vi "Orbitron2Websdr_MainApp_20032021.vi"() -> ()   [LabVIEW 2021]
uses:
  FHASOF_Groundstationsoftware/D/LabVIEW 2021/FHASOF_Groundstationsoftware/Multitrack.llb/Window Rectangle.ctl
  <vilib>/Utility/error.llb/whitespace.ctl
  <vilib>/Platform/TimedLoop/XDataNode/timing_clust.ctl
  <vilib>/Platform/TimedLoop/XDataNode/nitl_modes.ctl
  <vilib>/Platform/TimedLoop/XDataNode/wakeup.ctl
  <vilib>/Utility/error.llb/DialogType.ctl
  <vilib>/platform/TimedLoop/XDataNode/XDataNode.xnode
  <vilib>/Platform/TimedLoop/XDataNode/XDNodeRunTimeDep.lvlib
  <vilib>/Platform/browser.llb/Open URL in Default Browser (string).vi
panel:
  out "MaOps":bool
  out "error out 3":errorcluster
  out "error out 2":errorcluster
  out "path 3":path
  in  "Tab Control":T1(tab)
  out "Satellite Name":string
  in  "FocusCheck":bool
  in  "load":bool
  in  "Start browser":bool
  in  "preferences":bool
  in  "Stop_Button":bool
  out "Title 2":string="WebSDR Cat Control"
  in  "cw":bool
  in  "FocusWebSDR":bool
  in  "OpenWebSDR":bool
  in  "WebPages":u16(ring)=2 items=["IJsselstein, the Netherlands, JO22MA62KJ.", "IS0GRB VHF WebSDR Receiver IS0GRB / south sartinian iland", "Novovoronezh WebSDR WX"]
  in  "AddWebSDR":bool
  in  "Truncate Left digits":i32 caption="kHz"
  in  "Stop Cat Control":bool
  in  "Cat Control":bool
  in  "TaskList_Button":bool
  in  "processes Box":string(combo)="WebSDR on R3KEE in Novovoronezh - Google Chrome"
  out "Azimuth":string caption="°"
  out "Elevation":string caption="°"
  out "Downlink Freq.":string caption="KHz"
  in  "Downlink Freq. Man.":dbl=137100.0 caption="kHz" format="%#_6f"
  in  "ManualLatch":bool
  in  "Radio Mode":bool=TRUE
  in  "Type of DN":string
  in  "Downlink corr.":dbl(knob) scale=-100.0..100.0
  in  "USB":bool
  in  "LSB":bool
  in  "AM":bool
  in  "FM":bool
  in  "EditWebSDR":bool
  in  "DeleteWebSDR":bool
  out "Mode":string="Radio Manual mode"
  in  "Path of the webbrowser to start WebSDR":path=path "C:/Program Files/Google/Chrome/Application/chrome.exe"
  in  "goback_button":bool
  in  "Cancel Edit 2":bool
  out "data":string caption="DDE Message"
  in  "Sampling interval":u32=1000 caption="[ms]"
  in  "Load_button":bool
  in  "Cancel load":bool
  in  "Load controlfile":path=path "C:/Users/Setup/Documents/LabVIEW 2021"
  in  "Downlink corr.":string="0,000000"
  in  "Title":string="Add a new WebSDR database item"
  in  "Cancel Edit":bool
  in  "Edit_Button":bool
  in  "WebSDR Location / Name":string="Novovoronezh WebSDR WX"
  in  "Cancel Add":bool
  in  "Add_Button":bool
  in  "WebSDR URL":string="http://websdr.vrn.ru:8901/"
  in  "Window title":string="WebSDR on R3KEE in Novovoronezh - Google Chrome"
  in  "Truncate digits":string="2"
  out "Title 3":string="WebSDR Cat Control"
  in  "WebSDRDB":string[][](array[string])=[["IJsselstein, the Netherlands, JO22MA62KJ.", "WebSDR on Gerbrandy Tower in IJsselstein, NL - Google Chrome", "http://websdr.pi1utr.ampr.org:8901/", "0"], ["IS0GRB VHF WebSDR Receiver IS0GRB / south sartinian iland", "IS0GRB VHF WebSDR Receiver - Google Chrome", "http://websdr.is0grb.it:8902/", "2"], ["Novovoronezh WebSDR WX", "WebSDR on R3KEE in Novovoronezh - Google Chrome", "http://websdr.vrn.ru:8901/", "2"]]
  in  "Numeric":i32
  out "error out":errorcluster={"status"=FALSE, "code"=0, "source"="Get Window ID.vi"}
  out "Active Processses":string
  out "standard error":string
  out "standard output":string
  out "window rect 2":T2={"left"=-5, "top"=-564, "right"=1089, "bottom"=-2}
  in  "window names":string[](array[string])=["Orbitron 3.71", "WebSDR on R3KEE in Novovoronezh - Google Chrome", "Mydde", "RX-SSTV", "Task-Manager", "Einstellungen", "Einstellungen", "VIPM Service", "Microsoft Text Input Application", "Mail", "Posteingang – Hotmail ?- Mail", "Orbitron2Websdr_Win10Build", "RX-SSTV", "Program Manager", "LabVIEW"]
  in  "kill":bool
  in  "StopCatProgramatically":bool
  out "shutdown in":bool
  in  "iterCompleted":bool
  in  "slave4Killed":bool
  in  "slave3Killed":bool
  in  "slave1Killed":bool
  out "Elapsed Time (s)":dbl=3.000234603881836
  out "path 2":path
  out "path 4":path=path "C:/Users/Setup/Documents/LabVIEW 2021/Orbitron2Websdr_MainApp_20032021.ctr"
  out "path":path=path "C:/Users/Setup/Documents/LabVIEW 2021/Orbitron2Websdr_MainApp_20032021.ctr"
  out "concatenated string":string="Orbitron2Websdr_MainApp_20032021\\"
  out "string":string="C:\\Users\\Setup\\Documents\\LabVIEW 2021\\Orbitron2Websdr_MainApp_20032021.ctr"
  out "Parent Directory (+ Relative)":path=path "C:/Users/Setup/Documents/LabVIEW 2021"
  in  "dont write":bool
  in  "Interrupt":bool
  in  "AppName":string="WebSDR1"
  # "For Orbitron 3.71 MyDDE-Driver"
  # "To start WebSDR, you need a Webbrowser. We had good experiences using Firefox, so we selected Firefox as the default browser. If you want to start your WebSDR sessions with another browser,just select the executable of your preferred browser here:"
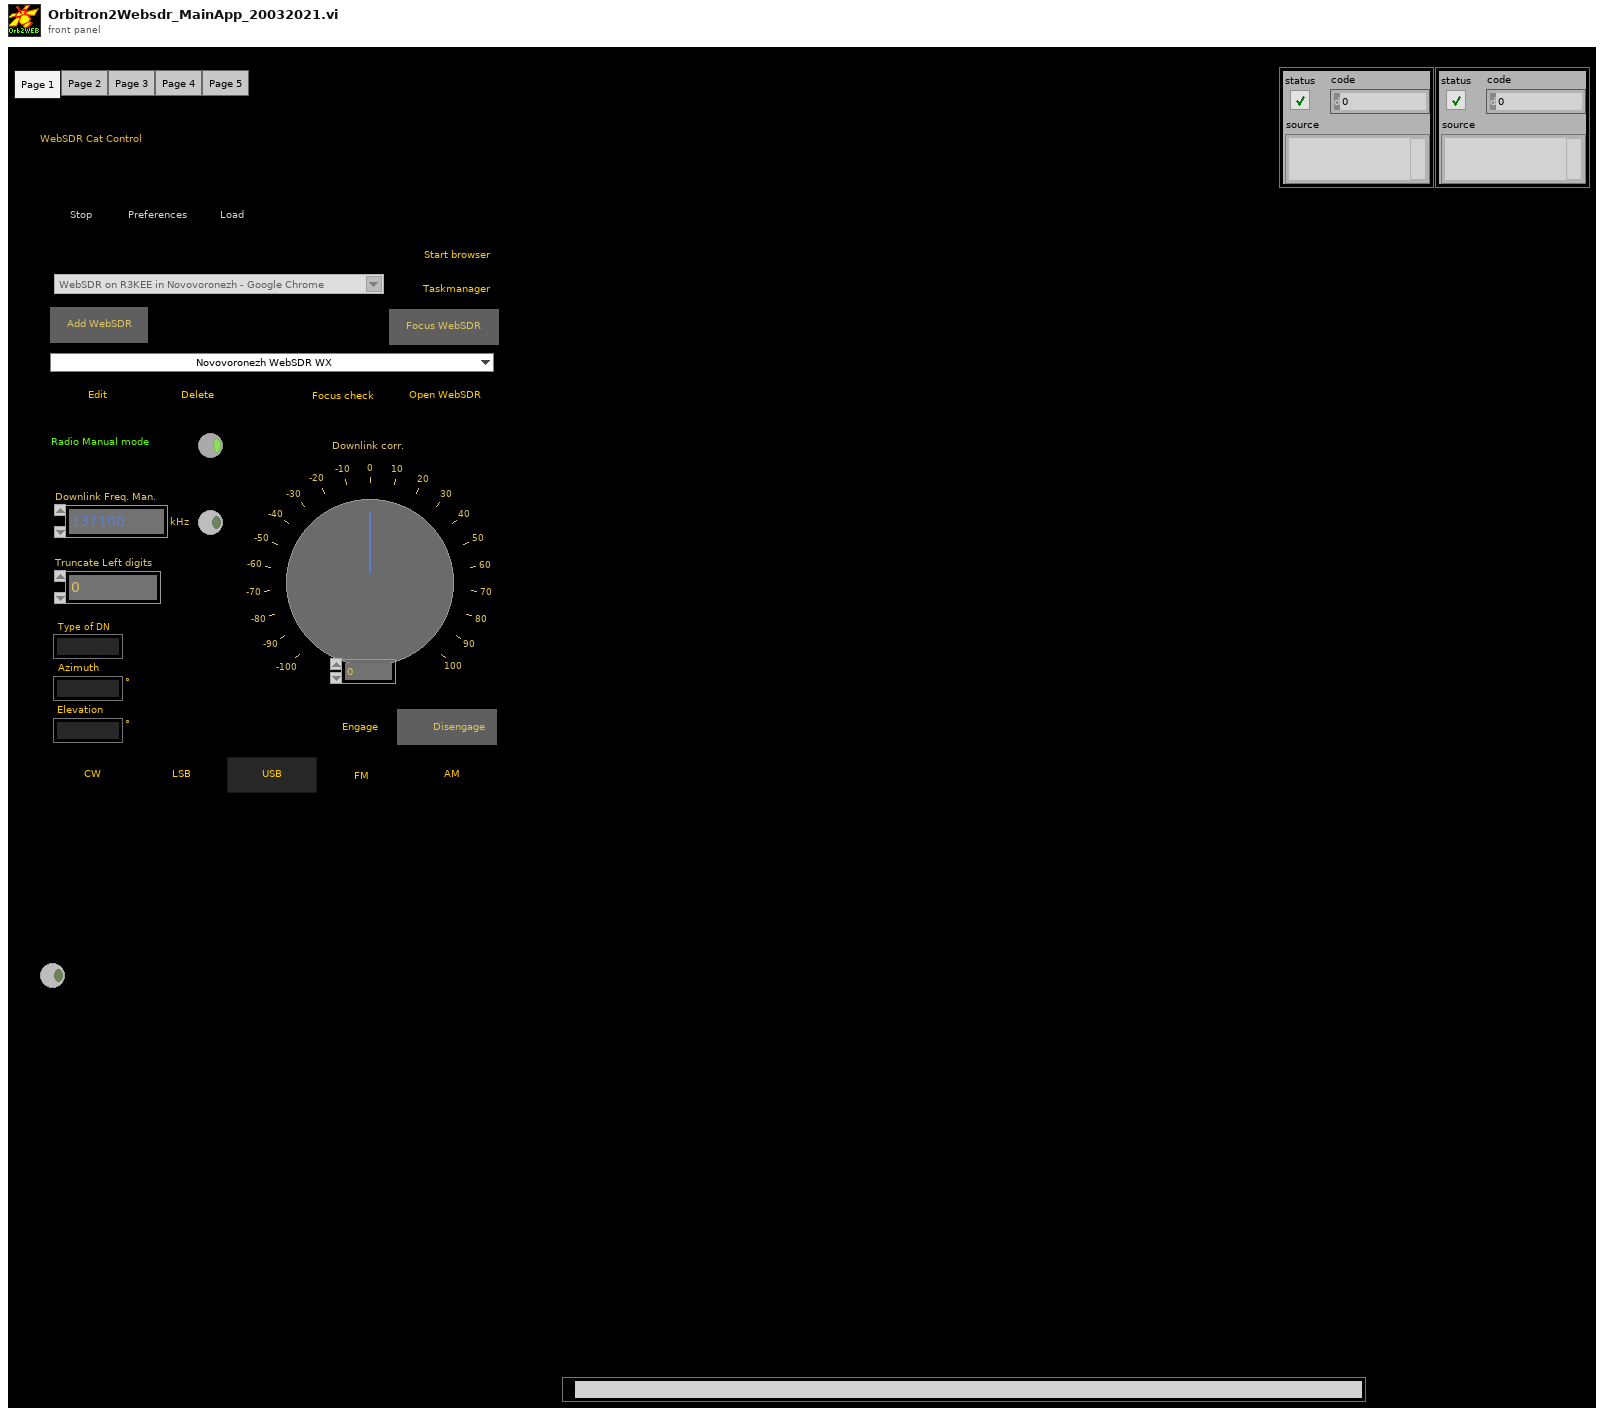
[diagram p1: front panel]
types:
  T1 = enum32{"Page 1", "Page 2", "Page 3", "Page 4", "Page 5"}
  T2 = typedef "Window Rectangle.ctl" = cluster{"left":i16, "top":i16, "right":i16, "bottom":i16}
  T3 = enum8{"Enabled", "Disabled", "Disabled and Grayed Out"}
  T4 = enum16{"Get Number of Tasks", "Get Window Info", "Get Window Names"}
  T5 = cluster{"number of windows":i32, "total names length":u32, "number of tasks found":i32, "window handles":u32[], "process ID":u32}
  T6 = typedef "Window Refnum" = refnum<k1>
  T7 = typedef "XDNodeRunTimeDep.lvlib/timing_clust.ctl" = cluster{"Expected End [f-1]":u64, "Actual End [f-1]":u64, "Finished Late? [f-1]":bool, "Expected End [i-1]":u64, "Actual End [i-1]":u64, "Finished Late? [i-1]":bool, "Expected Start [i]":u64, "Actual Start [i]":u64, "Expected Start [f]":u64, "Actual Start [f]":u64, "Source Name":string, "Structure Name":string, "Period":i64, "Deadline":i64, "Offset":i64, "Start":i64, "Priority":i32, "Timeout":i32, "Mode":T8, "Wakeup Reason":T9, "Error":errorcluster, "Source Type":string, "Secondary Source Type":string, "Global End Time":u64, "Global Start Time":u64, "Frame Duration":u64, "Iteration Duration":u64, "Assigned CPU":i32, "I/O Scan Engine Mode":u32}
  T8 = typedef "XDNodeRunTimeDep.lvlib/nitl_modes.ctl" = enum32{"No Change", "Process missed periods, maintain original phase", "Discard missed periods, maintain original phase", "Process missed periods, ignore original phase", "Discard missed periods, ignore original phase"}
  T9 = typedef "XDNodeRunTimeDep.lvlib/wakeup.ctl" = enum32{"Normal", "Aborted", "Asynchronous wakeup", "Timing source error", "Timed loop error", "Timeout"}
  T10 = typedef "DialogType.ctl" = u16
  T11 = typedef "whitespace.ctl" = u16
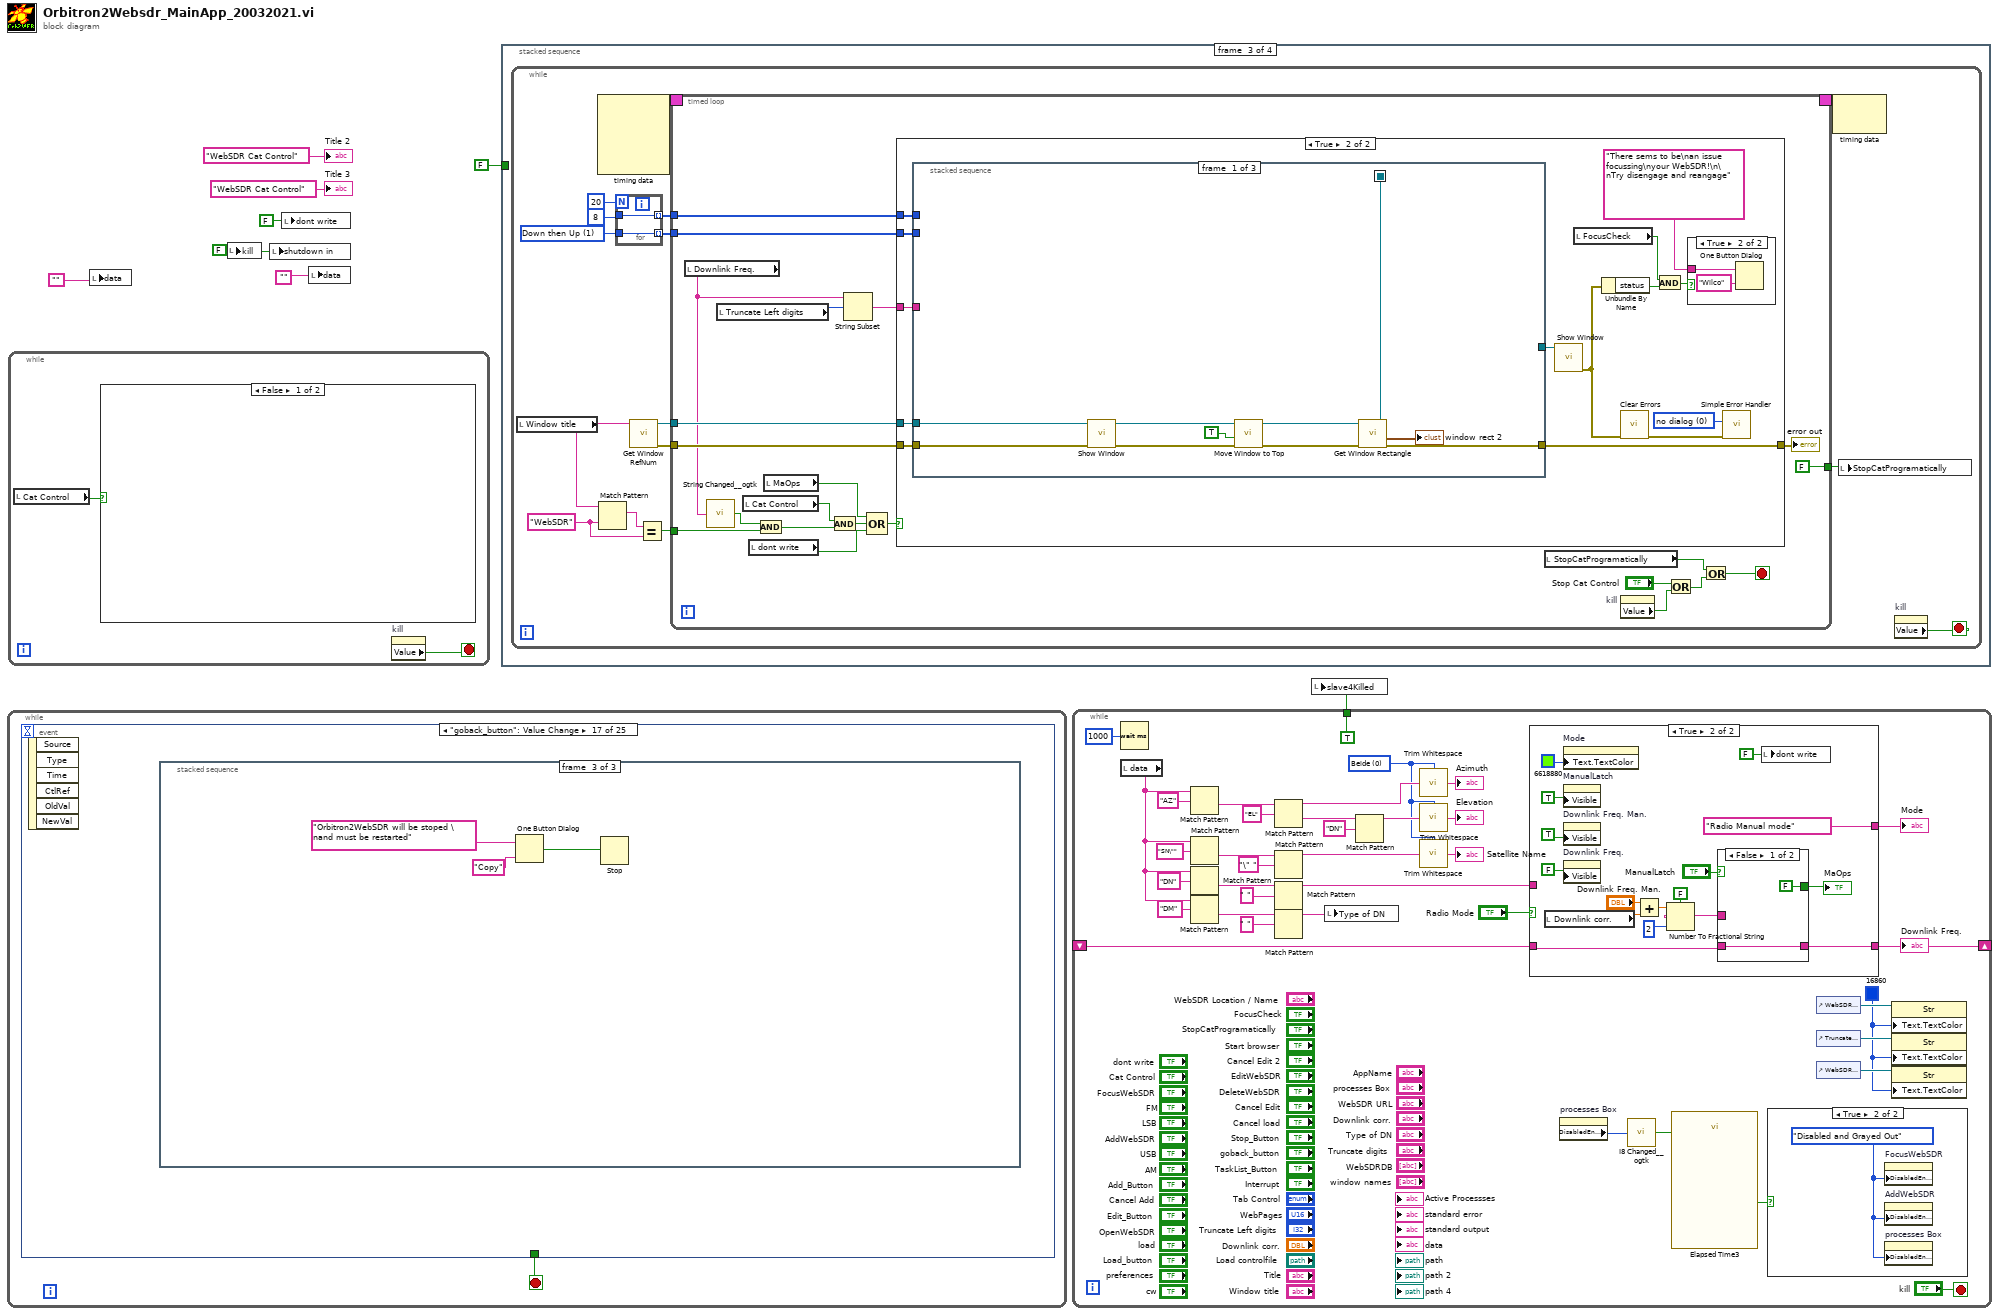
[diagram p0: block diagram]
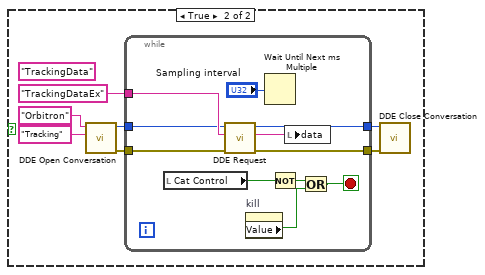
[diagram p2: hidden frame]
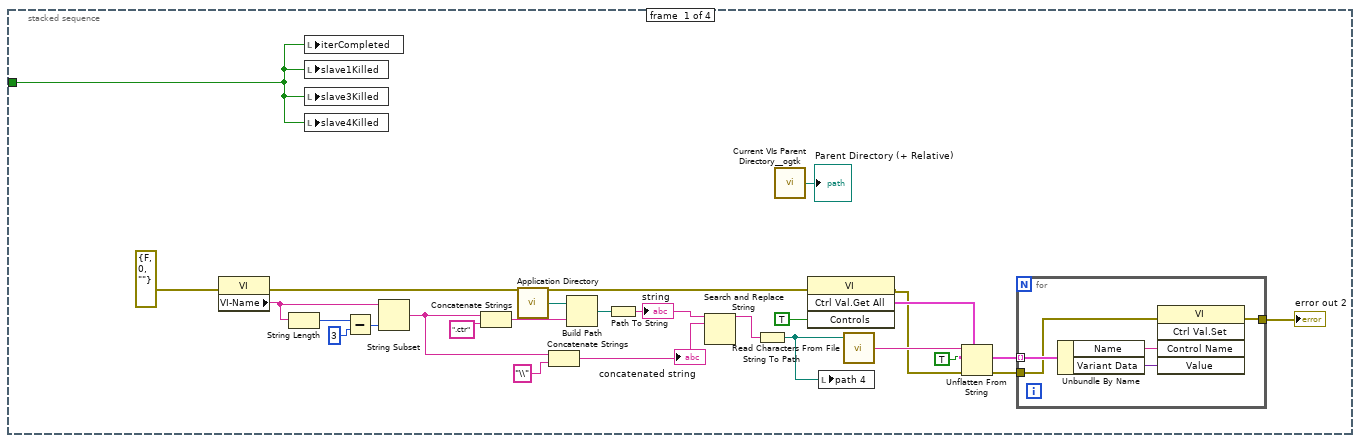
[diagram p3: hidden frame]
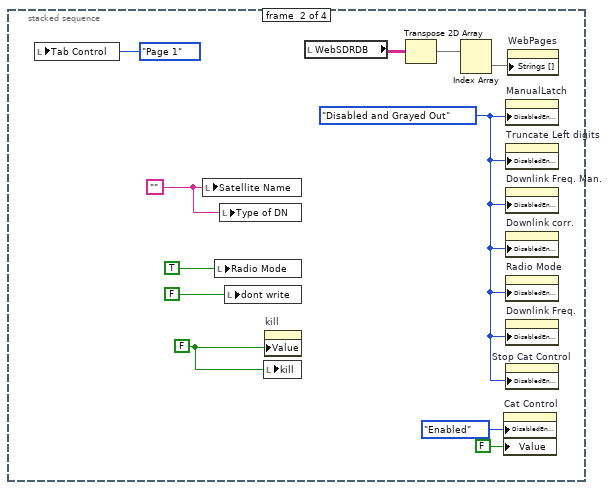
[diagram p4: hidden frame]
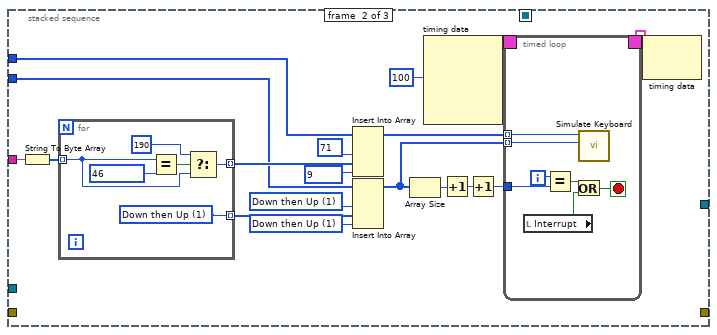
[diagram p7: hidden frame]
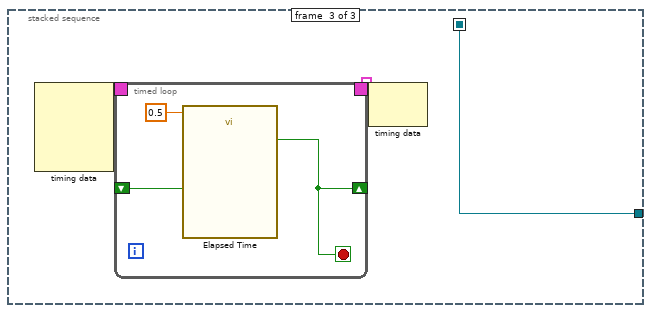
[diagram p8: hidden frame]
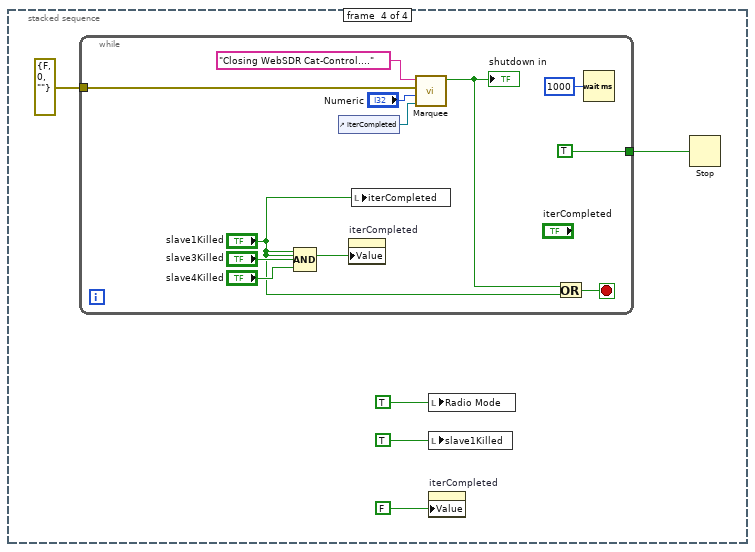
[diagram p9: hidden frame]
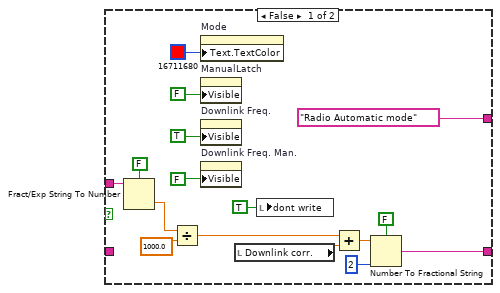
[diagram p11: hidden frame]
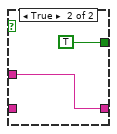
[diagram p12: hidden frame]
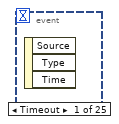
[diagram p13: hidden frame]
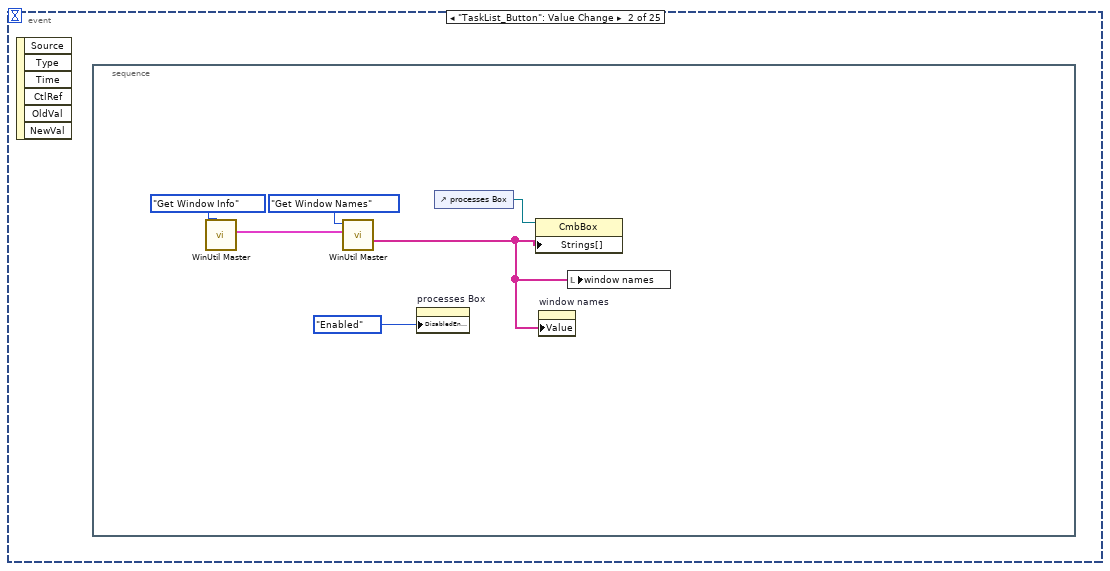
[diagram p14: hidden frame]
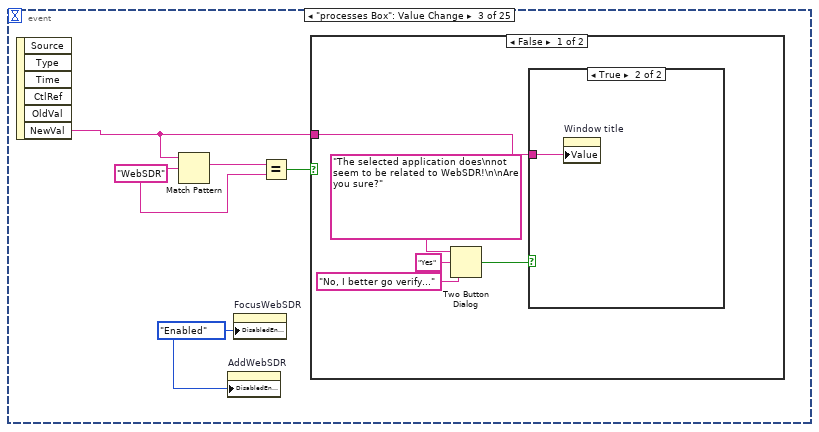
[diagram p15: hidden frame]
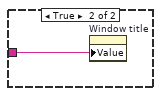
[diagram p17: hidden frame]
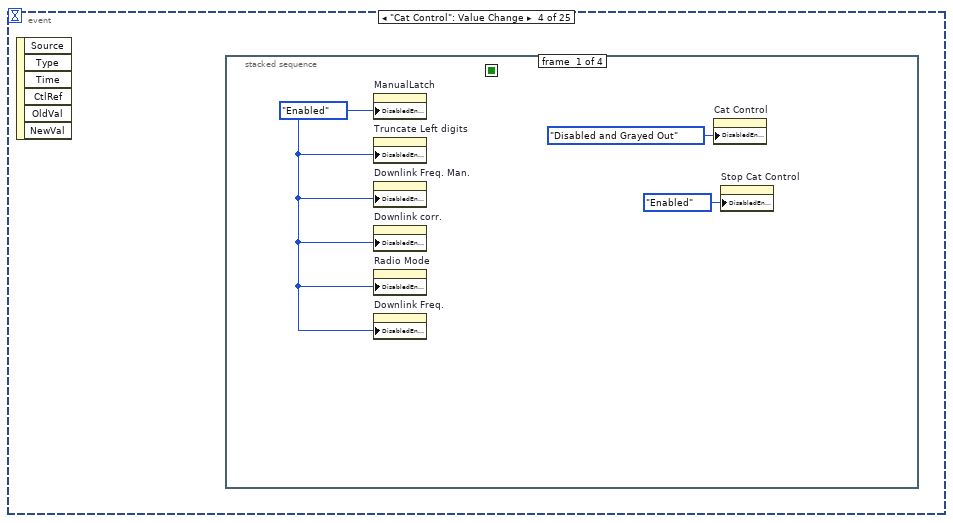
[diagram p18: hidden frame]
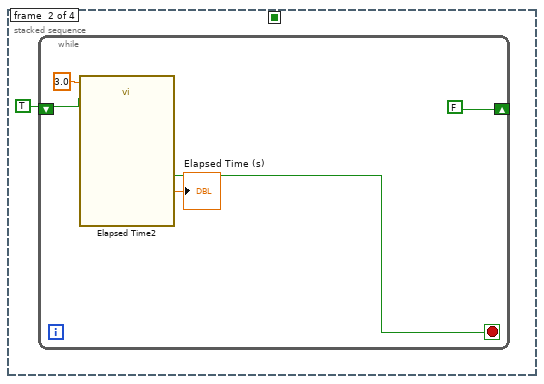
[diagram p19: hidden frame]
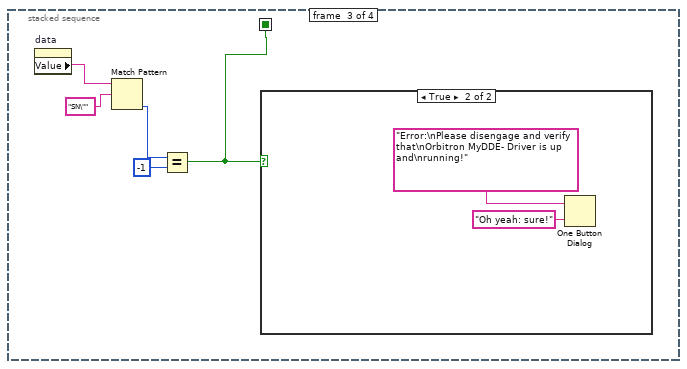
[diagram p20: hidden frame]
diagram:
  w6 = FALSE ("kill")
  n1 = while {
    stop <- w9 stop-if-true
    n2 = event shown="[16] \"goback_button\": Value Change" {
      selector: _ -> [_ _ _ _ _ _ _ _ _ _ _ _ _ _ _ _ _ _ _ _ _ _ _ _ _]
      dyn-events: _ -> [_ _ _ _ _ _ _ _ _ _ _ _ _ _ _ _ _ _ _ _ _ _ _ _ _]
      timeout: _ -> [_ _ _ _ _ _ _ _ _ _ _ _ _ _ _ _ _ _ _ _ _ _ _ _ _]
      tunnel: [_ _ _ _ w45 w95 _ _ _ _ _ _ _ _ _ _ _ _ _ _ _ _ _ _ _] -> w9
      event Timeout {
        n3 = event-data() -> ()  [unwired: 1 in, 3 out]
      }
      event "TaskList_Button": Value Change {
        n4 = event-data() -> ()  [unwired: 1 in, 6 out]
        n5 = stacked-sequence {
          frame #0 {
            n6 = call "WinUtil Master.vi"("function"=T4."Get Window Info") -> ("window enumeration info out"=w14:T5)  [unwired: 4 in, 2 out]
            n7 = call "WinUtil Master.vi"("window enumeration info in"=w14, "function"=T4."Get Window Names") -> ("window names"=w11:string[])  [unwired: 3 in, 2 out]
            n8 = property on="processes Box" class="CmbBox"("DisabledEnum"=T3."Enabled" ("Disabled")) -> ()  [unwired: 2 in, 2 out]
            n9 = control-ref of="processes Box"() -> (w15:refnum<vi>)
            n10 = property on="Property Node" class="CmbBox"(reference=w15, "Strings[]"=w11) -> ()  [unwired: 1 in, 2 out]
            n11 = property on="window names" class="Arr (strict)"("Value"=w11) -> ()  [unwired: 2 in, 2 out]
            n12 = local write "window names"(w11) -> ()
          }
        }
      }
      event "processes Box": Value Change {
        w17 = "WebSDR" ("Such-String")
        w20 = T3."Enabled" ("Disabled")
        n13 = event-data() -> ("NewVal"=w19:string)  [unwired: 1 in, 5 out]
        n14 = Match Pattern(string=w19, regular expression=w17) -> (match substring=w18:string)  [unwired: 1 in, 3 out]
        n15 = property on="AddWebSDR" class="Bool"("DisabledEnum"=w20) -> ()  [unwired: 2 in, 2 out]
        n16 = property on="FocusWebSDR" class="Bool"("DisabledEnum"=w20) -> ()  [unwired: 2 in, 2 out]
        n17 = Equal?(x=w18, y=w17) -> (x = y?=w16:bool)
        n18 = case shown="False" w16 {
          tunnel: w19 -> [w21 w27]
          frame False {
            n19 = Two Button Dialog(message="The selected application does\nnot seem to be related to WebSDR!\n\nAre you sure?", 1:"No, I better go verify..." ("F button name (\"Cancel\")"), 2:"Yes" ("T button name (\"OK\")")) -> (T button?=w22:bool)
            n20 = case shown="True" w22 {
              tunnel: w21 -> [_ w26]
              frame False {
              }
              frame True {
                n21 = property on="Window title" class="Str"("Value"=w26) -> ()  [unwired: 2 in, 2 out]
              }
            }
          }
          frame True {
            n22 = property on="Window title" class="Str"("Value"=w27) -> ()  [unwired: 2 in, 2 out]
          }
        }
      }
      event "Cat Control": Value Change {
        n23 = event-data() -> ()  [unwired: 1 in, 6 out]
        n24 = stacked-sequence {
          seq-local: [_ _ w38 _] -> [_ _ _ w44]
          frame #0 {
            w28 = T3."Enabled" ("Disabled")
            n25 = property on="ManualLatch" class="Bool"("DisabledEnum"=w28) -> ()  [unwired: 2 in, 2 out]
            n26 = property on="Truncate Left digits" class="DigNum (strict)"("DisabledEnum"=w28) -> ()  [unwired: 2 in, 2 out]
            n27 = property on="Downlink Freq. Man." class="DigNum (strict)"("DisabledEnum"=w28) -> ()  [unwired: 2 in, 2 out]
            n28 = property on="Downlink corr." class="Knob (strict)"("DisabledEnum"=w28) -> ()  [unwired: 2 in, 2 out]
            n29 = property on="Radio Mode" class="Bool (strict)"("DisabledEnum"=w28) -> ()  [unwired: 2 in, 2 out]
            n30 = property on="Downlink Freq." class="Str"("DisabledEnum"=w28) -> ()  [unwired: 2 in, 2 out]
            n31 = property on="Cat Control" class="Bool (strict)"("DisabledEnum"=T3."Disabled and Grayed Out" ("Disabled")) -> ()  [unwired: 2 in, 2 out]
            n32 = property on="Stop Cat Control" class="Bool"("DisabledEnum"=T3."Enabled" ("Disabled")) -> ()  [unwired: 2 in, 2 out]
          }
          frame #1 {
            n33 = while {
              shift-right: [FALSE] -> _
              shift-left: TRUE -> [w33]
              stop <- w35 stop-if-true
              n34 = call "Elapsed Time2"("Time Target (s)"=3.0, "Reset"=w33) -> ("Elapsed Time (s)"=→"Elapsed Time (s)":dbl, "Time has Elapsed"=w35:bool)  [unwired: 10 in, 6 out]
            }
          }
          frame #2 {
            n35 = property on="data" class="Str"() -> ("Value"=w37:string)  [unwired: 2 in, 2 out]
            n36 = Match Pattern(string=w37, regular expression="SN\"" ("Regulärer Ausdruck")) -> (offset past match=w40:i32)  [unwired: 1 in, 3 out]
            n37 = Equal?(x=w40, y=-1) -> (x = y?=w38:bool)
            n38 = case shown="True" w38 {
              frame False {
              }
              frame True {
                n39 = One Button Dialog(message="Error:\nPlease disengage and verify that\nOrbitron MyDDE- Driver is up and\nrunning!", button name ("OK")="Oh yeah: sure!") -> ()  [unwired: 1 out]
              }
            }
          }
          frame #3 {
            n40 = case shown="False" w44 {
              frame False {
                n41 = call "Display Message to User2"() -> ()  [unwired: 10 in, 2 out]
              }
              frame True {
              }
            }
          }
        }
      }
      event "Stop_Button": Value Change {
        n42 = event-data() -> ()  [unwired: 1 in, 6 out]
        n43 = stacked-sequence {
          tunnel: [_ _ w94] -> w45
          frame #0 {
            n44 = One Button Dialog(message="Ok WebSDR Cat Control\nwill be stoped!\nThis may take a while, \nso be a little bit patient!") -> ()  [unwired: 1 in, 1 out]
          }
          frame #1 {
            w55 = "websdrOrbitron" ("regular expression")
            n45 = property class="VI"() -> ("VI-Name"=w65:string)  [unwired: 2 in, 2 out]
            n46 = call "Current VIs Parent Directory__ogtk.vi"() -> ("Parent Directory (+ Relative)"=w49:path)  [unwired: 5 in]
            n47 = String Length(string=w65) -> (length=w63:i32)
            n48 = Subtract(x=w63, y=3) -> (x-y=w64:i32)
            n49 = String Subset(string=w65, length (rest)=w64) -> (substring=w82:string)  [unwired: 1 in]
            n50 = Concatenate Strings(w82, "*" ("string")) -> (w80:string)
            n51 = List Folder(path=w49, pattern=w80) -> (filenames=w81:string[])  [unwired: 2 in, 3 out]
            n52 = for {
              tunnel: w81 -> [w83] mode=indexing
              tunnel: w55 -> [w86]
              tunnel: [w85] -> w71 mode=indexing
              tunnel: [w83] -> _ mode=indexing
              n53 = Match Pattern(string=w83, regular expression=w86) -> (after substring=w84:string)  [unwired: 1 in, 3 out]
              n54 = Decimal String To Number(string=w84) -> (number=w85:i32)  [unwired: 2 in, 1 out]
            }
            n55 = Concatenate Strings(w82, ".ctr" ("String")) -> (w79:string)
            n56 = Build Path(base path=w49, name or relative path=w79) -> (appended path=w59:path)
            n57 = Array Max & Min(array=w71) -> (max value=w78:i32)  [unwired: 3 out]
            n58 = Concatenate Strings(w65, "\\" ("string")) -> (w62:string)
            n59 = Path To String(path=w59) -> (string=w60:string)
            n60 = Increment(x=w78) -> (x+1=w70:i32)
            n61 = Search and Replace String(input string=w60, search string=w62) -> (result string=w61:string)  [unwired: 6 in, 3 out]
            n62 = Format Value(format string="%03d", value (0)=w70) -> (output string=w69:string)  [unwired: 1 in]
            n63 = String To Path(string=w61) -> (path=w66:path)
            n64 = local write "path"(w66) -> ()
            n65 = Concatenate Strings(w55, w69) -> (w77:string)
            n66 = Concatenate Strings(w77, ".ctr" ("String")) -> (w72:string)
            n67 = invoke class="VI" method="Ctrl Val.Get All"("Controls"=TRUE ("controls")) -> ("Get All Control Values Variant"=w67:cluster{"Name":string, "Variant Data":variant}[])  [unwired: 3 in, 3 out]
            n68 = Build Path(base path=w49, name or relative path=w72) -> (appended path=w76:path)
            n69 = Concatenate Strings(w77, "\\" ("string")) -> (w73:string)
            n70 = Path To String(path=w76) -> (string=w75:string)
            n71 = Search and Replace String(input string=w75, search string=w73) -> (result string=w74:string)  [unwired: 6 in, 3 out]
            n72 = String To Path(string=w74) -> (path=w48:path)
            n73 = Flatten To String(anything=w67, prepend array or string size? (T)=TRUE) -> (data string=w68:string)  [unwired: 2 in, 2 out]
            n74 = stacked-sequence {
              tunnel: w66 -> [_ w89 _ w92 _]
              tunnel: w68 -> [w87 _ _ w91 _]
              tunnel: w48 -> [w88 _ _ _ _]
              frame #0 {
                n75 = call <vilib>:"Write Characters To File.vi"("character string"=w87, "file path (dialog if empty)"=w88) -> ()  [unwired: 3 in, 1 out]
              }
              frame #1 {
                n76 = Delete(path (use dialog)=w89) -> ()  [unwired: 4 in, 3 out]
              }
              frame #2 {
                n77 = Wait (ms)(milliseconds to wait=u32 2000) -> ()  [unwired: 1 out]
              }
              frame #3 {
                n78 = call <vilib>:"Write Characters To File.vi"("character string"=w91, "file path (dialog if empty)"=w92) -> ()  [unwired: 3 in, 1 out]
              }
              frame #4 {
                n79 = Wait (ms)(milliseconds to wait=u32 2000) -> ()  [unwired: 1 out]
              }
            }
          }
          frame #2 {
            w94 = TRUE ("kill")
            n80 = property on="kill" class="Bool (strict)"("Value"=w94) -> ()  [unwired: 2 in, 2 out]
          }
        }
      }
      event Panel Close? {
        n81 = event-data() -> ()  [unwired: 1 in, 4 out]
        n82 = stacked-sequence {
          tunnel: [_ _ _ w144] -> w95
          frame #0 {
            n83 = One Button Dialog(message="Ok WebSDR Cat Control\nwill be stoped!\nThis may take a while, \nso be a little bit patient!") -> ()  [unwired: 1 in, 1 out]
          }
          frame #1 {
            w104 = "websdrOrbitron" ("regular expression")
            n84 = property class="VI"() -> ("VI-Name"=w114:string)  [unwired: 2 in, 2 out]
            n85 = call "Current VIs Parent Directory__ogtk.vi"() -> ("Parent Directory (+ Relative)"=w126:path)  [unwired: 5 in]
            n86 = String Length(string=w114) -> (length=w112:i32)
            n87 = Subtract(x=w112, y=3) -> (x-y=w113:i32)
            n88 = String Subset(string=w114, length (rest)=w113) -> (substring=w132:string)  [unwired: 1 in]
            n89 = Concatenate Strings(w132, "*" ("string")) -> (w130:string)
            n90 = List Folder(path=w126, pattern=w130) -> (filenames=w131:string[])  [unwired: 2 in, 3 out]
            n91 = for {
              tunnel: w131 -> [w133] mode=indexing
              tunnel: w104 -> [w136]
              tunnel: [w135] -> w120 mode=indexing
              tunnel: [w133] -> _ mode=indexing
              n92 = Match Pattern(string=w133, regular expression=w136) -> (after substring=w134:string)  [unwired: 1 in, 3 out]
              n93 = Decimal String To Number(string=w134) -> (number=w135:i32)  [unwired: 2 in, 1 out]
            }
            n94 = Concatenate Strings(w132, ".ctr" ("String")) -> (w129:string)
            n95 = Build Path(base path=w126, name or relative path=w129) -> (appended path=w108:path)
            n96 = Array Max & Min(array=w120) -> (max value=w128:i32)  [unwired: 3 out]
            n97 = Concatenate Strings(w114, "\\" ("string")) -> (w111:string)
            n98 = Path To String(path=w108) -> (string=w109:string)
            n99 = Increment(x=w128) -> (x+1=w119:i32)
            n100 = Search and Replace String(input string=w109, search string=w111) -> (result string=w110:string)  [unwired: 6 in, 3 out]
            n101 = Format Value(format string="%03d", value (0)=w119) -> (output string=w118:string)  [unwired: 1 in]
            n102 = String To Path(string=w110) -> (path=w115:path)
            n103 = local write "path"(w115) -> ()
            n104 = Concatenate Strings(w104, w118) -> (w127:string)
            n105 = invoke class="VI" method="Ctrl Val.Get All"("Controls"=TRUE ("controls")) -> ("Get All Control Values Variant"=w116:cluster{"Name":string, "Variant Data":variant}[])  [unwired: 3 in, 3 out]
            n106 = Concatenate Strings(w127, ".ctr" ("String")) -> (w121:string)
            n107 = Build Path(base path=w126, name or relative path=w121) -> (appended path=w125:path)
            n108 = Concatenate Strings(w127, "\\" ("string")) -> (w122:string)
            n109 = Path To String(path=w125) -> (string=w124:string)
            n110 = Search and Replace String(input string=w124, search string=w122) -> (result string=w123:string)  [unwired: 6 in, 3 out]
            n111 = Flatten To String(anything=w116, prepend array or string size? (T)=TRUE) -> (data string=w117:string)  [unwired: 2 in, 2 out]
            n112 = String To Path(string=w123) -> (path=w98:path)
            n113 = stacked-sequence {
              tunnel: w115 -> [_ w139 _ w142 _]
              tunnel: w117 -> [w137 _ _ w141 _]
              tunnel: w98 -> [w138 _ _ _ _]
              frame #0 {
                n114 = call <vilib>:"Write Characters To File.vi"("character string"=w137, "file path (dialog if empty)"=w138) -> ()  [unwired: 3 in, 1 out]
              }
              frame #1 {
                n115 = Delete(path (use dialog)=w139) -> ()  [unwired: 4 in, 3 out]
              }
              frame #2 {
                n116 = Wait (ms)(milliseconds to wait=u32 4000) -> ()  [unwired: 1 out]
              }
              frame #3 {
                n117 = call <vilib>:"Write Characters To File.vi"("character string"=w141, "file path (dialog if empty)"=w142) -> ()  [unwired: 3 in, 1 out]
              }
              frame #4 {
                n118 = Wait (ms)(milliseconds to wait=u32 2000) -> ()  [unwired: 1 out]
              }
            }
            n119 = local write "path 2"(w98) -> ()
          }
          frame #2 {
          }
          frame #3 {
            w144 = TRUE ("kill")
            n120 = property on="kill" class="Bool (strict)"("Value"=w144) -> ()  [unwired: 2 in, 2 out]
          }
        }
        n121 = event-data("Discard?"=w95) -> ()  [unwired: 1 in, 1 out]
      }
      event "USB": Value Change {
        w150 = "WebSDR" ("Such-String")
        n122 = event-data() -> ()  [unwired: 1 in, 6 out]
        n123 = local read "Window title"() -> (w148:string)
        n124 = call "Get Window RefNum.vi"("window name (\"\")"=w148) -> ("error out"=w145:errorcluster, "window refnum (NaWR)"=w146:T6)  [unwired: 7 in]
        n125 = Match Pattern(string=w148, regular expression=w150) -> (match substring=w149:string)  [unwired: 1 in, 3 out]
        n126 = Equal?(x=w149, y=w150) -> (x = y?=w147:bool)
        n127 = case shown="True" w147 {
          tunnel: w146 -> [_ w155]
          tunnel: w145 -> [_ w154]
          frame False {
          }
          frame True {
            n128 = stacked-sequence {
              tunnel: w155 -> [w160 _]
              tunnel: w154 -> [w159 _]
              tunnel: [w158 _] -> w153
              tunnel: [w157 _] -> w152
              tunnel: [w156 _] -> w151
              frame #0 {
                n129 = call "Show Window.vi"("error in (no error)"=w159, "window refnum (NaWR)"=w160) -> ("window refnum out"=w163:T6)  [unwired: 4 in, 1 out]
                n130 = call "Move Window to Top.vi"("activate? (T)"=TRUE ("activate? (F)"), "window refnum (NaWR)"=w163) -> ("window refnum out"=w162:T6)  [unwired: 4 in, 1 out]
                n131 = call "Get Window Rectangle.vi"("window refnum (NaWR)"=w162) -> ("error out"=w157:errorcluster, "window rect"=w156:T2, "window refnum out"=w158:T6)  [unwired: 4 in]
              }
              frame #1 {
                w164 = u32 1 items=["Down/Press", "Down then Up", "Up/Release"] ("Action")
                n132 = call "Simulate Keyboard.vi"("Action"=w164, "Virtual Key"=u8 85) -> ()  [unwired: 7 in, 1 out]
              }
            }
            n133 = local write "window rect 2"(w151) -> ()
            n134 = call "Show Window.vi"("error in (no error)"=w152, "window refnum (NaWR)"=w153) -> ()  [unwired: 4 in, 2 out]
          }
        }
      }
      event "cw": Value Change {
        w171 = "WebSDR" ("Such-String")
        n135 = event-data() -> ()  [unwired: 1 in, 6 out]
        n136 = local read "Window title"() -> (w169:string)
        n137 = call "Get Window RefNum.vi"("window name (\"\")"=w169) -> ("error out"=w166:errorcluster, "window refnum (NaWR)"=w167:T6)  [unwired: 7 in]
        n138 = Match Pattern(string=w169, regular expression=w171) -> (match substring=w170:string)  [unwired: 1 in, 3 out]
        n139 = Equal?(x=w170, y=w171) -> (x = y?=w168:bool)
        n140 = case shown="True" w168 {
          tunnel: w167 -> [_ w176]
          tunnel: w166 -> [_ w175]
          frame False {
          }
          frame True {
            n141 = stacked-sequence {
              tunnel: w176 -> [w181 _]
              tunnel: w175 -> [w180 _]
              tunnel: [w179 _] -> w174
              tunnel: [w178 _] -> w173
              tunnel: [w177 _] -> w172
              frame #0 {
                n142 = call "Show Window.vi"("error in (no error)"=w180, "window refnum (NaWR)"=w181) -> ("window refnum out"=w184:T6)  [unwired: 4 in, 1 out]
                n143 = call "Move Window to Top.vi"("activate? (T)"=TRUE ("activate? (F)"), "window refnum (NaWR)"=w184) -> ("window refnum out"=w183:T6)  [unwired: 4 in, 1 out]
                n144 = call "Get Window Rectangle.vi"("window refnum (NaWR)"=w183) -> ("error out"=w178:errorcluster, "window rect"=w177:T2, "window refnum out"=w179:T6)  [unwired: 4 in]
              }
              frame #1 {
                w185 = u32 1 items=["Down/Press", "Down then Up", "Up/Release"] ("Action")
                n145 = call "Simulate Keyboard.vi"("Action"=w185, "Virtual Key"=u8 67) -> ()  [unwired: 7 in, 1 out]
              }
            }
            n146 = local write "window rect 2"(w172) -> ()
            n147 = call "Show Window.vi"("error in (no error)"=w173, "window refnum (NaWR)"=w174) -> ()  [unwired: 4 in, 2 out]
          }
        }
      }
      event "LSB": Value Change {
        w192 = "WebSDR" ("Such-String")
        n148 = event-data() -> ()  [unwired: 1 in, 6 out]
        n149 = local read "Window title"() -> (w190:string)
        n150 = call "Get Window RefNum.vi"("window name (\"\")"=w190) -> ("error out"=w187:errorcluster, "window refnum (NaWR)"=w188:T6)  [unwired: 7 in]
        n151 = Match Pattern(string=w190, regular expression=w192) -> (match substring=w191:string)  [unwired: 1 in, 3 out]
        n152 = Equal?(x=w191, y=w192) -> (x = y?=w189:bool)
        n153 = case shown="True" w189 {
          tunnel: w188 -> [_ w197]
          tunnel: w187 -> [_ w196]
          frame False {
          }
          frame True {
            n154 = stacked-sequence {
              tunnel: w197 -> [w202 _]
              tunnel: w196 -> [w201 _]
              tunnel: [w200 _] -> w195
              tunnel: [w199 _] -> w194
              tunnel: [w198 _] -> w193
              frame #0 {
                n155 = call "Show Window.vi"("error in (no error)"=w201, "window refnum (NaWR)"=w202) -> ("window refnum out"=w205:T6)  [unwired: 4 in, 1 out]
                n156 = call "Move Window to Top.vi"("activate? (T)"=TRUE ("activate? (F)"), "window refnum (NaWR)"=w205) -> ("window refnum out"=w204:T6)  [unwired: 4 in, 1 out]
                n157 = call "Get Window Rectangle.vi"("window refnum (NaWR)"=w204) -> ("error out"=w199:errorcluster, "window rect"=w198:T2, "window refnum out"=w200:T6)  [unwired: 4 in]
              }
              frame #1 {
                w206 = u32 1 items=["Down/Press", "Down then Up", "Up/Release"] ("Action")
                n158 = call "Simulate Keyboard.vi"("Action"=w206, "Virtual Key"=u8 76) -> ()  [unwired: 7 in, 1 out]
              }
            }
            n159 = local write "window rect 2"(w193) -> ()
            n160 = call "Show Window.vi"("error in (no error)"=w194, "window refnum (NaWR)"=w195) -> ()  [unwired: 4 in, 2 out]
          }
        }
      }
      event "FM": Value Change {
        w213 = "WebSDR" ("Such-String")
        n161 = event-data() -> ()  [unwired: 1 in, 6 out]
        n162 = local read "Window title"() -> (w211:string)
        n163 = call "Get Window RefNum.vi"("window name (\"\")"=w211) -> ("error out"=w208:errorcluster, "window refnum (NaWR)"=w209:T6)  [unwired: 7 in]
        n164 = Match Pattern(string=w211, regular expression=w213) -> (match substring=w212:string)  [unwired: 1 in, 3 out]
        n165 = Equal?(x=w212, y=w213) -> (x = y?=w210:bool)
        n166 = case shown="True" w210 {
          tunnel: w209 -> [_ w218]
          tunnel: w208 -> [_ w217]
          frame False {
          }
          frame True {
            n167 = stacked-sequence {
              tunnel: w218 -> [w223 _]
              tunnel: w217 -> [w222 _]
              tunnel: [w221 _] -> w216
              tunnel: [w220 _] -> w215
              tunnel: [w219 _] -> w214
              frame #0 {
                n168 = call "Show Window.vi"("error in (no error)"=w222, "window refnum (NaWR)"=w223) -> ("window refnum out"=w226:T6)  [unwired: 4 in, 1 out]
                n169 = call "Move Window to Top.vi"("activate? (T)"=TRUE ("activate? (F)"), "window refnum (NaWR)"=w226) -> ("window refnum out"=w225:T6)  [unwired: 4 in, 1 out]
                n170 = call "Get Window Rectangle.vi"("window refnum (NaWR)"=w225) -> ("error out"=w220:errorcluster, "window rect"=w219:T2, "window refnum out"=w221:T6)  [unwired: 4 in]
              }
              frame #1 {
                w227 = u32 1 items=["Down/Press", "Down then Up", "Up/Release"] ("Action")
                n171 = call "Simulate Keyboard.vi"("Action"=w227, "Virtual Key"=u8 70) -> ()  [unwired: 7 in, 1 out]
              }
            }
            n172 = local write "window rect 2"(w214) -> ()
            n173 = call "Show Window.vi"("error in (no error)"=w215, "window refnum (NaWR)"=w216) -> ()  [unwired: 4 in, 2 out]
          }
        }
      }
      event "AM": Value Change {
        w234 = "WebSDR" ("Such-String")
        n174 = event-data() -> ()  [unwired: 1 in, 6 out]
        n175 = local read "Window title"() -> (w232:string)
        n176 = call "Get Window RefNum.vi"("window name (\"\")"=w232) -> ("error out"=w229:errorcluster, "window refnum (NaWR)"=w230:T6)  [unwired: 7 in]
        n177 = Match Pattern(string=w232, regular expression=w234) -> (match substring=w233:string)  [unwired: 1 in, 3 out]
        n178 = Equal?(x=w233, y=w234) -> (x = y?=w231:bool)
        n179 = case shown="True" w231 {
          tunnel: w230 -> [_ w239]
          tunnel: w229 -> [_ w238]
          frame False {
          }
          frame True {
            n180 = stacked-sequence {
              tunnel: w239 -> [w244 _]
              tunnel: w238 -> [w243 _]
              tunnel: [w242 _] -> w237
              tunnel: [w241 _] -> w236
              tunnel: [w240 _] -> w235
              frame #0 {
                n181 = call "Show Window.vi"("error in (no error)"=w243, "window refnum (NaWR)"=w244) -> ("window refnum out"=w247:T6)  [unwired: 4 in, 1 out]
                n182 = call "Move Window to Top.vi"("activate? (T)"=TRUE ("activate? (F)"), "window refnum (NaWR)"=w247) -> ("window refnum out"=w246:T6)  [unwired: 4 in, 1 out]
                n183 = call "Get Window Rectangle.vi"("window refnum (NaWR)"=w246) -> ("error out"=w241:errorcluster, "window rect"=w240:T2, "window refnum out"=w242:T6)  [unwired: 4 in]
              }
              frame #1 {
                w248 = u32 1 items=["Down/Press", "Down then Up", "Up/Release"] ("Action")
                n184 = call "Simulate Keyboard.vi"("Action"=w248, "Virtual Key"=u8 65) -> ()  [unwired: 7 in, 1 out]
              }
            }
            n185 = local write "window rect 2"(w235) -> ()
            n186 = call "Show Window.vi"("error in (no error)"=w236, "window refnum (NaWR)"=w237) -> ()  [unwired: 4 in, 2 out]
          }
        }
      }
      event "OpenWebSDR": Value Change {
        n187 = event-data() -> ()  [unwired: 1 in, 6 out]
        n188 = stacked-sequence {
          frame #0 {
            n189 = while {
              stop <- w251 stop-if-true
              n190 = call "You selected a WebSDR- site for your Satellite-operations"() -> ("OK"=w251:bool)  [unwired: 18 in, 1 out]
              n191 = Wait (ms)(milliseconds to wait=u32 500) -> ()  [unwired: 1 out]
            }
          }
          frame #1 {
            (unwired) "C:\\Program Files\\Mozilla Firefox\\firefox.exe "
            n192 = disable-structure shown="Disabled" {
              frame Disabled {
                n193 = call-poly <vilib>:"Open URL in Default Browser.vi"("URL"="http://websdr.is0grb.it:8902/") -> ()  [unwired: 5 in, 2 out]
              }
              frame Enabled {
              }
            }
            n194 = local read "WebSDRDB"() -> (w269:string[][])
            n195 = Transpose 2D Array(2D array=w269) -> (transposed array=w270:string[][])
            n196 = local read "Path of the webbrowser to start WebSDR"() -> (w255:path)
            n197 = Index Array(array=w270, index (row) #1=1 ("index (row)"), index (row) #2=2 ("index (row)"), index (row) #3=3 ("index (row)")) -> (element #1=w260:string[], element #2=w268:string[], element #3=w263:string[])  [unwired: 3 in]
            n198 = property on="WebPages" class="Ring (strict)"() -> ("Value"=w259:u16)  [unwired: 2 in, 2 out]
            n199 = Index Array(array=w260, index=w259) -> (element=w258:string)
            n200 = Index Array(array=w268, index=w259) -> (element=w253:string)
            n201 = Index Array(array=w263, index=w259) -> (element=w262:string)
            n202 = Path To String(path=w255) -> (string=w254:string)
            n203 = Decimal String To Number(string=w262) -> (number=w264:i32)  [unwired: 2 in, 1 out]
            n204 = Concatenate Strings(w254, " " ("string"), w253) -> (w266:string)
            n205 = local write "Truncate Left digits"(w264) -> ()
            n206 = local write "Window title"(w258) -> ()
            n207 = call <vilib>:"System Exec.vi"("wait until completion? (T)"=FALSE, "command line"=w266) -> ("standard error"=w257:string, "standard output"=w256:string)  [unwired: 6 in, 2 out]
            n208 = local write "standard output"(w256) -> ()
            n209 = local write "standard error"(w257) -> ()
          }
        }
      }
      event "Start browser": Value Change {
        (unwired) "C:\\Program Files\\Mozilla Firefox\\firefox.exe "
        n210 = event-data() -> ()  [unwired: 1 in, 6 out]
        n211 = local read "Path of the webbrowser to start WebSDR"() -> (w276:path)
        n212 = Path To String(path=w276) -> (string=w275:string)
        n213 = Concatenate Strings(w275, " ", "http://websdr.org" ("URL")) -> (w277:string)
        n214 = call <vilib>:"System Exec.vi"("command line"=w277) -> ("standard error"=w279:string, "standard output"=w278:string)  [unwired: 7 in, 2 out]
        n215 = local write "standard output"(w278) -> ()
        n216 = local write "standard error"(w279) -> ()
      }
      event "preferences": Value Change {
        n217 = event-data() -> ()  [unwired: 1 in, 6 out]
        n218 = local write "Tab Control"(T1."Page 2" ("Tab Control")) -> ()
      }
      event "load": Value Change {
        n219 = event-data() -> ()  [unwired: 1 in, 6 out]
        n220 = local write "Tab Control"(T1."Page 3" ("Tab Control")) -> ()
        n221 = call "Current VIs Parent Directory__ogtk.vi"() -> ("Parent Directory (+ Relative)"=w281:path)  [unwired: 5 in]
        n222 = local write "Load controlfile"(w281) -> ()
      }
      event "Load_button": Value Change {
        n223 = event-data() -> ()  [unwired: 1 in, 6 out]
        n224 = stacked-sequence {
          frame #0 {
            n225 = local read "Load controlfile"() -> (w284:path)
            n226 = invoke class="VI" method="Ctrl Val.Get All"(error in=errorcluster {"status"=FALSE, "code"=0, "source"=""} ("error in (no error)"), "Controls"=TRUE) -> (error out=w292:errorcluster, "Get All Control Values Variant"=w289:cluster{"Name":string, "Variant Data":variant}[])  [unwired: 2 in, 2 out]
            n227 = call <vilib>:"Read Characters From File.vi"("file path (dialog if empty)"=w284) -> ("character string"=w285:string)  [unwired: 5 in, 3 out]
            n228 = Unflatten From String(type=w289, binary string=w285, data includes array or string size? (T)=TRUE, error in (no error)=w292) -> (value=w287:cluster{"Name":string, "Variant Data":variant}[], error out=w290:errorcluster)  [unwired: 1 in, 1 out]
            n229 = for {
              tunnel: w287 -> [w297] mode=indexing
              tunnel: w290 -> [w294]
              tunnel: [w293] -> w291
              n230 = Unbundle By Name(w297) -> ("Name"=w295:string, "Variant Data"=w296:variant)
              n231 = invoke class="VI" method="Ctrl Val.Set"(error in=w294, "Control Name"=w295, "Value"=w296) -> (error out=w293:errorcluster)  [unwired: 2 in, 4 out]
            }
            "error out 3" <- w291
          }
          frame #1 {
            n232 = local write "Tab Control"(T1."Page 1" ("Tab Control")) -> ()
          }
        }
      }
      event "goback_button": Value Change {
        n233 = event-data() -> ()  [unwired: 1 in, 6 out]
        n234 = stacked-sequence {
          frame #0 {
            w304 = "websdr" ("regular expression")
            n235 = property class="VI"() -> ("VI-Name"=w314:string)  [unwired: 2 in, 2 out]
            n236 = call "Current VIs Parent Directory__ogtk.vi"() -> ("Parent Directory (+ Relative)"=w326:path)  [unwired: 5 in]
            n237 = String Length(string=w314) -> (length=w312:i32)
            n238 = Subtract(x=w312, y=3) -> (x-y=w313:i32)
            n239 = String Subset(string=w314, length (rest)=w313) -> (substring=w333:string)  [unwired: 1 in]
            n240 = Concatenate Strings(w333, "*" ("string")) -> (w331:string)
            n241 = List Folder(path=w326, pattern=w331) -> (filenames=w332:string[])  [unwired: 2 in, 3 out]
            n242 = for {
              tunnel: w332 -> [w334] mode=indexing
              tunnel: w304 -> [w337]
              tunnel: [w336] -> w320 mode=indexing
              tunnel: [w334] -> _ mode=indexing
              n243 = Match Pattern(string=w334, regular expression=w337) -> (after substring=w335:string)  [unwired: 1 in, 3 out]
              n244 = Decimal String To Number(string=w335) -> (number=w336:i32)  [unwired: 2 in, 1 out]
            }
            n245 = Concatenate Strings(w333, ".ctr" ("String")) -> (w330:string)
            n246 = Build Path(base path=w326, name or relative path=w330) -> (appended path=w308:path)
            n247 = Array Max & Min(array=w320) -> (max value=w329:i32)  [unwired: 3 out]
            n248 = Concatenate Strings(w314, "\\" ("string")) -> (w311:string)
            n249 = Path To String(path=w308) -> (string=w309:string)
            n250 = Increment(x=w329) -> (x+1=w319:i32)
            n251 = Search and Replace String(input string=w309, search string=w311) -> (result string=w310:string)  [unwired: 6 in, 3 out]
            n252 = Format Value(format string="%03d", value (0)=w319) -> (output string=w318:string)  [unwired: 1 in]
            n253 = String To Path(string=w310) -> (path=w315:path)
            "path 3" <- w315
            n254 = local write "path"(w315) -> ()
            n255 = Concatenate Strings(w304, w318) -> (w328:string)
            n256 = Concatenate Strings(w328, ".ctr" ("String")) -> (w321:string)
            n257 = invoke class="VI" method="Ctrl Val.Get All"("Controls"=TRUE ("controls")) -> ("Get All Control Values Variant"=w316:cluster{"Name":string, "Variant Data":variant}[])  [unwired: 3 in, 3 out]
            n258 = Build Path(base path=w326, name or relative path=w321) -> (appended path=w325:path)
            n259 = Concatenate Strings(w328, "\\" ("string")) -> (w322:string)
            n260 = Path To String(path=w325) -> (string=w324:string)
            n261 = Search and Replace String(input string=w324, search string=w322) -> (result string=w323:string)  [unwired: 6 in, 3 out]
            n262 = Flatten To String(anything=w316) -> (data string=w317:string)  [unwired: 3 in, 2 out]
            n263 = String To Path(string=w323) -> (path=w327:path)
            n264 = stacked-sequence {
              tunnel: w315 -> [_ w340 _ w343 _]
              tunnel: w317 -> [w338 _ _ w342 _]
              tunnel: w327 -> [w339 _ _ _ _]
              frame #0 {
                n265 = call <vilib>:"Write Characters To File.vi"("character string"=w338, "file path (dialog if empty)"=w339) -> ()  [unwired: 3 in, 1 out]
              }
              frame #1 {
                n266 = Delete(path (use dialog)=w340) -> ()  [unwired: 4 in, 3 out]
              }
              frame #2 {
                n267 = Wait (ms)(milliseconds to wait=u32 2000) -> ()  [unwired: 1 out]
              }
              frame #3 {
                n268 = call <vilib>:"Write Characters To File.vi"("character string"=w342, "file path (dialog if empty)"=w343) -> ()  [unwired: 3 in, 1 out]
              }
              frame #4 {
                n269 = Wait (ms)(milliseconds to wait=u32 2000) -> ()  [unwired: 1 out]
              }
            }
          }
          frame #1 {
            n270 = local write "Tab Control"(T1."Page 1" ("Tab Control")) -> ()
          }
          frame #2 {
            n271 = One Button Dialog(message="Orbitron2WebSDR will be stoped \nand must be restarted", button name ("OK")="Copy") -> (true=w346:bool)
            n272 = Stop(stop? (T)=w346) -> ()
          }
        }
      }
      event "FocusWebSDR": Value Change {
        n273 = event-data() -> ()  [unwired: 1 in, 6 out]
        n274 = flat-sequence {
          frame #0 {
            n275 = property on="processes Box" class="CmbBox"() -> ("Text.Text"=w354:string)  [unwired: 2 in, 2 out]
            n276 = local write "Window title"(w354) -> ()
            n277 = call "Get Window RefNum.vi"("window name (\"\")"=w354) -> ("error out"=w350:errorcluster, "window refnum (NaWR)"=w351:T6)  [unwired: 7 in]
            n278 = call "Show Window.vi"("error in (no error)"=w350, "window refnum (NaWR)"=w351) -> ("error out"=w353:errorcluster, "window refnum out"=w352:T6)  [unwired: 4 in]
            n279 = call "Move Window to Top.vi"("error in (no error)"=w353, "activate? (T)"=TRUE ("activate? (F)"), "window refnum (NaWR)"=w352) -> ()  [unwired: 3 in, 2 out]
          }
          frame #1 {
            n280 = call "You selected a WebSDR- site for your Satellite-operations2"() -> ()  [unwired: 18 in, 2 out]
          }
        }
      }
      event "AddWebSDR": Value Change {
        w357 = ""
        w360 = FALSE
        w359 = TRUE
        n281 = event-data() -> ()  [unwired: 1 in, 6 out]
        n282 = local read "Truncate Left digits"() -> (w362:i32)
        n283 = local read "Downlink corr."() -> (w356:dbl)
        n284 = local write "WebSDR Location / Name"(w357) -> ()
        n285 = local write "Tab Control"(enum32{"Page 1", "Page 2", "Page 3", "Page 4"}."Page 4" ("Tab Control")) -> ()
        n286 = Number To Fractional String(number=w356) -> (F-format string=w355:string)  [unwired: 3 in]
        n287 = local write "WebSDR URL"(w357) -> ()
        n288 = Number To Decimal String(number=w362) -> (decimal integer string=w361:string)  [unwired: 1 in]
        n289 = local write "Downlink corr."(w355) -> ()
        n290 = local write "Truncate digits"(w361) -> ()
        n291 = local write "Title"("Add a new WebSDR database item" ("Title")) -> ()
        n292 = property on="Cancel Add" class="Bool"("Visible"=w359) -> ()  [unwired: 2 in, 2 out]
        n293 = property on="Add_Button" class="Bool"("Visible"=w359) -> ()  [unwired: 2 in, 2 out]
        n294 = property on="Cancel Edit" class="Bool"("Visible"=w360) -> ()  [unwired: 2 in, 2 out]
        n295 = property on="Edit_Button" class="Bool"("Visible"=w360) -> ()  [unwired: 2 in, 2 out]
      }
      event "Add_Button": Value Change {
        n296 = event-data() -> ()  [unwired: 1 in, 6 out]
        n297 = stacked-sequence {
          frame #0 {
            n298 = local read "WebSDR Location / Name"() -> (w369:string)
            n299 = local read "WebSDRDB"() -> (w373:string[][])
            n300 = local read "WebSDR URL"() -> (w365:string)
            n301 = local read "Window title"() -> (w372:string)
            n302 = local read "Downlink corr."() -> (w364:string)
            n303 = local read "Truncate digits"() -> (w370:string)
            n304 = Build Array(w369, w372, w365, w370, w364) -> (w371:string[])
            n305 = Insert Into Array(array=w373, new element=w371) -> (w367:string[][])  [unwired: 2 in]
            n306 = local write "WebSDRDB"(w367) -> ()
            n307 = Transpose 2D Array(2D array=w367) -> (transposed array=w366:string[][])
            n308 = Index Array(array=w366) -> (element=w368:string[])  [unwired: 2 in]
            n309 = property on="WebPages" class="Ring (strict)"("Strings []"=w368) -> ()  [unwired: 2 in, 2 out]
          }
          frame #1 {
            n310 = local write "Tab Control"(enum32{"Page 1", "Page 2", "Page 3", "Page 4"}."Page 1" ("Tab Control")) -> ()
            n311 = property on="WebPages" class="Ring (strict)"("Value"=0) -> ()  [unwired: 2 in, 2 out]
          }
          frame #2 {
            w392 = "websdrOrbitron" ("regular expression")
            n312 = property class="VI"() -> ("VI-Name"=w387:string)  [unwired: 2 in, 2 out]
            n313 = String Length(string=w387) -> (length=w382:i32)
            n314 = call "Current VIs Parent Directory__ogtk.vi"() -> ("Parent Directory (+ Relative)"=w407:path)  [unwired: 5 in]
            n315 = Subtract(x=w382, y=3) -> (x-y=w384:i32)
            n316 = String Subset(string=w387, length (rest)=w384) -> (substring=w397:string)  [unwired: 1 in]
            n317 = Concatenate Strings(w397, "*" ("string")) -> (w399:string)
            n318 = List Folder(path=w407, pattern=w399) -> (filenames=w376:string[])  [unwired: 2 in, 3 out]
            n319 = for {
              tunnel: w376 -> [w414] mode=indexing
              tunnel: w392 -> [w413]
              tunnel: [w411] -> w396 mode=indexing
              n320 = Match Pattern(string=w414, regular expression=w413) -> (after substring=w412:string)  [unwired: 1 in, 3 out]
              n321 = Decimal String To Number(string=w412) -> (number=w411:i32)  [unwired: 2 in, 1 out]
            }
            n322 = Concatenate Strings(w397, ".ctr" ("String")) -> (w386:string)
            n323 = Build Path(base path=w407, name or relative path=w386) -> (appended path=w377:path)
            n324 = Concatenate Strings(w387, "\\" ("string")) -> (w381:string)
            n325 = Array Max & Min(array=w396) -> (max value=w410:i32)  [unwired: 3 out]
            n326 = Path To String(path=w377) -> (string=w378:string)
            n327 = Increment(x=w410) -> (x+1=w395:i32)
            n328 = Search and Replace String(input string=w378, search string=w381) -> (result string=w379:string)  [unwired: 6 in, 3 out]
            n329 = String To Path(string=w379) -> (path=w388:path)
            n330 = Format Value(format string="%03d", value (0)=w395) -> (output string=w393:string)  [unwired: 1 in]
            n331 = local write "path"(w388) -> ()
            n332 = Concatenate Strings(w392, w393) -> (w409:string)
            n333 = Concatenate Strings(w409, ".ctr" ("String")) -> (w400:string)
            n334 = Build Path(base path=w407, name or relative path=w400) -> (appended path=w406:path)
            n335 = Concatenate Strings(w409, "\\" ("string")) -> (w402:string)
            n336 = invoke class="VI" method="Ctrl Val.Get All"("Controls"=TRUE ("controls")) -> ("Get All Control Values Variant"=w389:cluster{"Name":string, "Variant Data":variant}[])  [unwired: 3 in, 3 out]
            n337 = Path To String(path=w406) -> (string=w405:string)
            n338 = Search and Replace String(input string=w405, search string=w402) -> (result string=w404:string)  [unwired: 6 in, 3 out]
            n339 = String To Path(string=w404) -> (path=w408:path)
            n340 = Flatten To String(anything=w389) -> (data string=w391:string)  [unwired: 3 in, 2 out]
            n341 = stacked-sequence {
              tunnel: w388 -> [_ w417 w419]
              tunnel: w391 -> [w415 _ w418]
              tunnel: w408 -> [w416 _ _]
              frame #0 {
                n342 = call <vilib>:"Write Characters To File.vi"("character string"=w415, "file path (dialog if empty)"=w416) -> ()  [unwired: 3 in, 1 out]
              }
              frame #1 {
                n343 = Delete(path (use dialog)=w417) -> ()  [unwired: 4 in, 3 out]
              }
              frame #2 {
                n344 = call <vilib>:"Write Characters To File.vi"("character string"=w418, "file path (dialog if empty)"=w419) -> ()  [unwired: 3 in, 1 out]
              }
            }
          }
        }
      }
      event "Edit_Button": Value Change {
        n345 = event-data() -> ()  [unwired: 1 in, 6 out]
        n346 = stacked-sequence {
          frame #0 {
            n347 = local read "WebSDR Location / Name"() -> (w427:string)
            n348 = local read "WebSDRDB"() -> (w430:string[][])
            n349 = local read "WebSDR URL"() -> (w423:string)
            n350 = local read "Window title"() -> (w429:string)
            n351 = local read "Downlink corr."() -> (w420:string)
            n352 = local read "Truncate digits"() -> (w428:string)
            n353 = property on="WebPages" class="Ring (strict)"() -> ("Value"=w422:u16)  [unwired: 2 in, 2 out]
            n354 = Build Array(w427, w429, w423, w428, w420) -> (w421:string[])
            n355 = Replace Array Subset(array=w430, new element=w421, index (row)=w422) -> (w425:string[][])  [unwired: 1 in]
            n356 = Transpose 2D Array(2D array=w425) -> (transposed array=w424:string[][])
            n357 = local write "WebSDRDB"(w425) -> ()
            n358 = Index Array(array=w424) -> (element=w426:string[])  [unwired: 2 in]
            n359 = property on="WebPages" class="Ring (strict)"("Strings []"=w426) -> ()  [unwired: 2 in, 2 out]
          }
          frame #1 {
            n360 = local write "Tab Control"(enum32{"Page 1", "Page 2", "Page 3", "Page 4"}."Page 1" ("Tab Control")) -> ()
            n361 = property on="WebPages" class="Ring (strict)"("Value"=0) -> ()  [unwired: 2 in, 2 out]
          }
          frame #2 {
            w449 = "websdrOrbitron" ("regular expression")
            n362 = property class="VI"() -> ("VI-Name"=w444:string)  [unwired: 2 in, 2 out]
            n363 = String Length(string=w444) -> (length=w439:i32)
            n364 = call "Current VIs Parent Directory__ogtk.vi"() -> ("Parent Directory (+ Relative)"=w464:path)  [unwired: 5 in]
            n365 = Subtract(x=w439, y=3) -> (x-y=w441:i32)
            n366 = String Subset(string=w444, length (rest)=w441) -> (substring=w454:string)  [unwired: 1 in]
            n367 = Concatenate Strings(w454, "*" ("string")) -> (w456:string)
            n368 = List Folder(path=w464, pattern=w456) -> (filenames=w433:string[])  [unwired: 2 in, 3 out]
            n369 = for {
              tunnel: w433 -> [w471] mode=indexing
              tunnel: w449 -> [w470]
              tunnel: [w468] -> w453 mode=indexing
              n370 = Match Pattern(string=w471, regular expression=w470) -> (after substring=w469:string)  [unwired: 1 in, 3 out]
              n371 = Decimal String To Number(string=w469) -> (number=w468:i32)  [unwired: 2 in, 1 out]
            }
            n372 = Concatenate Strings(w454, ".ctr" ("String")) -> (w443:string)
            n373 = Build Path(base path=w464, name or relative path=w443) -> (appended path=w434:path)
            n374 = Concatenate Strings(w444, "\\" ("string")) -> (w438:string)
            n375 = Array Max & Min(array=w453) -> (max value=w467:i32)  [unwired: 3 out]
            n376 = Path To String(path=w434) -> (string=w435:string)
            n377 = Increment(x=w467) -> (x+1=w452:i32)
            n378 = Search and Replace String(input string=w435, search string=w438) -> (result string=w436:string)  [unwired: 6 in, 3 out]
            n379 = String To Path(string=w436) -> (path=w445:path)
            n380 = Format Value(format string="%03d", value (0)=w452) -> (output string=w450:string)  [unwired: 1 in]
            n381 = local write "path"(w445) -> ()
            n382 = Concatenate Strings(w449, w450) -> (w466:string)
            n383 = Concatenate Strings(w466, ".ctr" ("String")) -> (w457:string)
            n384 = Build Path(base path=w464, name or relative path=w457) -> (appended path=w463:path)
            n385 = Concatenate Strings(w466, "\\" ("string")) -> (w459:string)
            n386 = invoke class="VI" method="Ctrl Val.Get All"("Controls"=TRUE ("controls")) -> ("Get All Control Values Variant"=w446:cluster{"Name":string, "Variant Data":variant}[])  [unwired: 3 in, 3 out]
            n387 = Path To String(path=w463) -> (string=w462:string)
            n388 = Search and Replace String(input string=w462, search string=w459) -> (result string=w461:string)  [unwired: 6 in, 3 out]
            n389 = String To Path(string=w461) -> (path=w465:path)
            n390 = Flatten To String(anything=w446) -> (data string=w448:string)  [unwired: 3 in, 2 out]
            n391 = stacked-sequence {
              tunnel: w445 -> [_ w474 w476]
              tunnel: w448 -> [w472 _ w475]
              tunnel: w465 -> [w473 _ _]
              frame #0 {
                n392 = call <vilib>:"Write Characters To File.vi"("character string"=w472, "file path (dialog if empty)"=w473) -> ()  [unwired: 3 in, 1 out]
              }
              frame #1 {
                n393 = Delete(path (use dialog)=w474) -> ()  [unwired: 4 in, 3 out]
              }
              frame #2 {
                n394 = call <vilib>:"Write Characters To File.vi"("character string"=w475, "file path (dialog if empty)"=w476) -> ()  [unwired: 3 in, 1 out]
              }
            }
          }
        }
      }
      event "DeleteWebSDR": Value Change {
        n395 = event-data() -> ()  [unwired: 1 in, 6 out]
        n396 = property on="WebPages" class="Ring (strict)"() -> ("RingText.Text"=w478:string)  [unwired: 2 in, 2 out]
        n397 = Concatenate Strings("Are you sure to delete the Mode specification:\n" ("message"), w478, "?" ("string")) -> (w483:string)
        n398 = Two Button Dialog(message=w483, 1:"No" ("F button name (\"Cancel\")"), 2:"Yes" ("T button name (\"OK\")")) -> (T button?=w477:bool)
        n399 = case shown="True" w477 {
          frame False {
          }
          frame True {
            n400 = stacked-sequence {
              frame #0 {
                n401 = local read "WebSDRDB"() -> (w486:string[][])
                n402 = property on="WebPages" class="Ring (strict)"() -> ("Value"=w484:u16)  [unwired: 2 in, 2 out]
                n403 = Delete From Array(array=w486, index (row)=w484) -> (array with subset deleted=w485:string[][])  [unwired: 2 in, 1 out]
                n404 = local write "WebSDRDB"(w485) -> ()
              }
              frame #1 {
                n405 = property on="WebPages" class="Ring (strict)"("Value"=0) -> ()  [unwired: 2 in, 2 out]
                n406 = local write "Tab Control"(enum32{"Page 1", "Page 2", "Page 3", "Page 4"}."Page 1" ("Tab Control")) -> ()
              }
              frame #2 {
                w505 = "websdrOrbitron" ("regular expression")
                n407 = property class="VI"() -> ("VI-Name"=w500:string)  [unwired: 2 in, 2 out]
                n408 = String Length(string=w500) -> (length=w495:i32)
                n409 = call "Current VIs Parent Directory__ogtk.vi"() -> ("Parent Directory (+ Relative)"=w520:path)  [unwired: 5 in]
                n410 = Subtract(x=w495, y=3) -> (x-y=w497:i32)
                n411 = String Subset(string=w500, length (rest)=w497) -> (substring=w510:string)  [unwired: 1 in]
                n412 = Concatenate Strings(w510, "*" ("string")) -> (w512:string)
                n413 = List Folder(path=w520, pattern=w512) -> (filenames=w489:string[])  [unwired: 2 in, 3 out]
                n414 = for {
                  tunnel: w489 -> [w527] mode=indexing
                  tunnel: w505 -> [w526]
                  tunnel: [w524] -> w509 mode=indexing
                  n415 = Match Pattern(string=w527, regular expression=w526) -> (after substring=w525:string)  [unwired: 1 in, 3 out]
                  n416 = Decimal String To Number(string=w525) -> (number=w524:i32)  [unwired: 2 in, 1 out]
                }
                n417 = Concatenate Strings(w510, ".ctr" ("String")) -> (w499:string)
                n418 = Build Path(base path=w520, name or relative path=w499) -> (appended path=w490:path)
                n419 = Concatenate Strings(w500, "\\" ("string")) -> (w494:string)
                n420 = Array Max & Min(array=w509) -> (max value=w523:i32)  [unwired: 3 out]
                n421 = Path To String(path=w490) -> (string=w491:string)
                n422 = Increment(x=w523) -> (x+1=w508:i32)
                n423 = Search and Replace String(input string=w491, search string=w494) -> (result string=w492:string)  [unwired: 6 in, 3 out]
                n424 = String To Path(string=w492) -> (path=w501:path)
                n425 = Format Value(format string="%03d", value (0)=w508) -> (output string=w506:string)  [unwired: 1 in]
                n426 = local write "path"(w501) -> ()
                n427 = Concatenate Strings(w505, w506) -> (w522:string)
                n428 = Concatenate Strings(w522, ".ctr" ("String")) -> (w513:string)
                n429 = Build Path(base path=w520, name or relative path=w513) -> (appended path=w519:path)
                n430 = Concatenate Strings(w522, "\\" ("string")) -> (w515:string)
                n431 = invoke class="VI" method="Ctrl Val.Get All"("Controls"=TRUE ("controls")) -> ("Get All Control Values Variant"=w502:cluster{"Name":string, "Variant Data":variant}[])  [unwired: 3 in, 3 out]
                n432 = Path To String(path=w519) -> (string=w518:string)
                n433 = Search and Replace String(input string=w518, search string=w515) -> (result string=w517:string)  [unwired: 6 in, 3 out]
                n434 = String To Path(string=w517) -> (path=w521:path)
                n435 = Flatten To String(anything=w502) -> (data string=w504:string)  [unwired: 3 in, 2 out]
                n436 = stacked-sequence {
                  tunnel: w501 -> [_ w530 w532]
                  tunnel: w504 -> [w528 _ w531]
                  tunnel: w521 -> [w529 _ _]
                  frame #0 {
                    n437 = call <vilib>:"Write Characters To File.vi"("character string"=w528, "file path (dialog if empty)"=w529) -> ()  [unwired: 3 in, 1 out]
                  }
                  frame #1 {
                    n438 = Delete(path (use dialog)=w530) -> ()  [unwired: 4 in, 3 out]
                  }
                  frame #2 {
                    n439 = call <vilib>:"Write Characters To File.vi"("character string"=w531, "file path (dialog if empty)"=w532) -> ()  [unwired: 3 in, 1 out]
                  }
                }
              }
            }
          }
        }
      }
      event "Cancel load", "Cancel Edit", "Cancel Edit 2": Value Change {
        n440 = event-data() -> ()  [unwired: 1 in, 6 out]
        n441 = local write "Tab Control"(enum32{"Page 1", "Page 2", "Page 3", "Page 4"}."Page 1" ("Tab Control")) -> ()
      }
      event "EditWebSDR": Value Change {
        w534 = TRUE
        w536 = FALSE
        n442 = event-data() -> ()  [unwired: 1 in, 6 out]
        n443 = local read "WebSDRDB"() -> (w550:string[][])
        n444 = Transpose 2D Array(2D array=w550) -> (transposed array=w551:string[][])
        n445 = local write "Tab Control"(enum32{"Page 1", "Page 2", "Page 3", "Page 4"}."Page 4" ("Tab Control")) -> ()
        n446 = Index Array(array=w551, index (row) #1=0 ("index (row)"), index (row) #2=1 ("index (row)"), index (row) #3=2 ("index (row)"), index (row) #4=3 ("index (row)")) -> (element #1=w541:string[], element #2=w547:string[], element #3=w549:string[], element #4=w548:string[])  [unwired: 4 in]
        n447 = local write "Title"("Edit WebSDR database item" ("Title")) -> ()
        n448 = property on="WebPages" class="Ring (strict)"() -> ("Value"=w542:u16)  [unwired: 2 in, 2 out]
        n449 = Index Array(array=w541, index=w542) -> (element=w540:string)
        n450 = Index Array(array=w547, index=w542) -> (element=w539:string)
        n451 = Index Array(array=w549, index=w542) -> (element=w538:string)
        n452 = Index Array(array=w548, index=w542) -> (element=w537:string)
        n453 = local write "WebSDR Location / Name"(w540) -> ()
        n454 = local write "Window title"(w539) -> ()
        n455 = local write "WebSDR URL"(w538) -> ()
        n456 = local write "Truncate digits"(w537) -> ()
        n457 = property on="Cancel Add" class="Bool"("Visible"=w536) -> ()  [unwired: 2 in, 2 out]
        n458 = property on="Add_Button" class="Bool"("Visible"=w536) -> ()  [unwired: 2 in, 2 out]
        n459 = property on="Cancel Edit" class="Bool"("Visible"=w534) -> ()  [unwired: 2 in, 2 out]
        n460 = property on="Edit_Button" class="Bool"("Visible"=w534) -> ()  [unwired: 2 in, 2 out]
      }
      event "Stop Cat Control": Value Change {
        w553 = ""
        w555 = TRUE
        w556 = T3."Disabled and Grayed Out" ("Disabled")
        n461 = event-data() -> ()  [unwired: 1 in, 6 out]
        n462 = local write "dont write"(FALSE ("dont write")) -> ()
        n463 = local write "Radio Mode"(w555) -> ()
        n464 = property on="Radio Mode" class="Bool (strict)"("Value"=w555) -> ()  [unwired: 2 in, 2 out]
        n465 = property on="Cat Control" class="Bool (strict)"("DisabledEnum"=T3."Enabled" ("Disabled"), "Value"=FALSE ("Cat Control")) -> ()  [unwired: 2 in, 2 out]
        n466 = property on="ManualLatch" class="Bool"("DisabledEnum"=w556) -> ()  [unwired: 2 in, 2 out]
        n467 = property on="Truncate Left digits" class="DigNum (strict)"("DisabledEnum"=w556) -> ()  [unwired: 2 in, 2 out]
        n468 = property on="Downlink Freq. Man." class="DigNum (strict)"("DisabledEnum"=w556) -> ()  [unwired: 2 in, 2 out]
        n469 = property on="Downlink corr." class="Knob (strict)"("DisabledEnum"=w556) -> ()  [unwired: 2 in, 2 out]
        n470 = property on="Radio Mode" class="Bool (strict)"("DisabledEnum"=w556) -> ()  [unwired: 2 in, 2 out]
        n471 = property on="Downlink Freq." class="Str"("DisabledEnum"=w556) -> ()  [unwired: 2 in, 2 out]
        n472 = property on="Stop Cat Control" class="Bool"("DisabledEnum"=T3."Disabled and Grayed Out" ("Disabled")) -> ()  [unwired: 2 in, 2 out]
        n473 = local write "data"(w553) -> ()
        n474 = property on="data" class="Str"("Value"=w553) -> ()  [unwired: 2 in, 2 out]
      }
    }
  }
  n475 = while {
    stop <- w561 stop-if-true
    n476 = local read "Cat Control"() -> (w560:bool)
    n477 = case shown="False" w560 {
      frame False {
      }
      frame True {
        (unwired) "TrackingData" ("item")
        n478 = call "DDE Open Conversation.vi"("topic"="Tracking" ("Topic"), "service"="Orbitron" ("Service")) -> ("error out"=w565:errorcluster, "conversation refnum"=w566:u32)  [unwired: 6 in]
        n479 = while {
          tunnel: w566 -> [w578]
          tunnel: w565 -> [w577]
          tunnel: "TrackingDataEx" ("item") -> [w579]
          tunnel: [w576] -> w564
          tunnel: [w575] -> w563
          stop <- w570 stop-if-true
          n480 = local read "Cat Control"() -> (w573:bool)
          n481 = call "DDE Request.vi"("error in (no error)"=w577, "item"=w579, "conversation refnum in"=w578) -> ("error out"=w575:errorcluster, "data"=w572:string, "conversation refnum out"=w576:u32)  [unwired: 4 in]
          n482 = property on="kill" class="Bool (strict)"() -> ("Value"=w569:bool)  [unwired: 2 in, 2 out]
          n483 = Wait Until Next ms Multiple(millisecond multiple="Sampling interval") -> ()  [unwired: 1 out]
          n484 = Not(x=w573) -> (.not. x?=w571:bool)
          n485 = local write "data"(w572) -> ()
          n486 = Or(x=w571, y=w569) -> (x .or. y?=w570:bool)
        }
        n487 = call "DDE Close Conversation.vi"("error in (no error)"=w563, "conversation refnum"=w564) -> ()  [unwired: 7 in, 1 out]
      }
    }
    n488 = property on="kill" class="Bool (strict)"() -> ("Value"=w561:bool)  [unwired: 2 in, 2 out]
  }
  n489 = local write "data"("") -> ()
  n490 = local write "kill"(w6) -> ()
  n491 = local write "shutdown in"(w6) -> ()
  n492 = local write "dont write"(FALSE ("dont write")) -> ()
  n493 = local write "data"("") -> ()
  n494 = stacked-sequence {
    tunnel: FALSE ("iterCompleted") -> [w594 _ _ _]
    frame #0 {
      n495 = property class="VI"(error in=errorcluster {"status"=FALSE, "code"=0, "source"=""} ("error in (no error)")) -> (error out=w583:errorcluster, "VI-Name"=w602:string)  [unwired: 1 in, 1 out]
      n496 = String Length(string=w602) -> (length=w600:i32)
      n497 = local write "iterCompleted"(w594) -> ()
      n498 = local write "slave1Killed"(w594) -> ()
      n499 = local write "slave3Killed"(w594) -> ()
      n500 = local write "slave4Killed"(w594) -> ()
      n501 = Subtract(x=w600, y=3) -> (x-y=w598:i32)
      n502 = String Subset(string=w602, length (rest)=w598) -> (substring=w595:string)  [unwired: 1 in]
      n503 = Concatenate Strings(w595, ".ctr" ("String")) -> (w596:string)
      n504 = call <vilib>:"Application Directory.vi"() -> ("Application Directory"=w581:path)
      n505 = Concatenate Strings(w595, "\\" ("string")) -> (w592:string)
      "concatenated string" <- w592
      n506 = Build Path(base path=w581, name or relative path=w596) -> (appended path=w593:path)
      n507 = Path To String(path=w593) -> (string=w591:string)
      "string" <- w591
      n508 = Search and Replace String(input string=w591, search string=w592) -> (result string=w590:string)  [unwired: 6 in, 3 out]
      n509 = String To Path(string=w590) -> (path=w589:path)
      n510 = call "Current VIs Parent Directory__ogtk.vi"() -> ("Parent Directory (+ Relative)"=→"Parent Directory (+ Relative)":path)  [unwired: 5 in]
      n511 = invoke class="VI" method="Ctrl Val.Get All"(error in=w583, "Controls"=TRUE) -> (error out=w582:errorcluster, "Get All Control Values Variant"=w587:cluster{"Name":string, "Variant Data":variant}[])  [unwired: 2 in, 2 out]
      n512 = local write "path 4"(w589) -> ()
      n513 = call <vilib>:"Read Characters From File.vi"("file path (dialog if empty)"=w589) -> ("character string"=w605:string)  [unwired: 5 in, 3 out]
      n514 = Unflatten From String(type=w587, binary string=w605, data includes array or string size? (T)=TRUE, error in (no error)=w582) -> (value=w603:cluster{"Name":string, "Variant Data":variant}[], error out=w586:errorcluster)  [unwired: 1 in, 1 out]
      n515 = for {
        tunnel: w603 -> [w610] mode=indexing
        tunnel: w586 -> [w607]
        tunnel: [w606] -> w585
        n516 = Unbundle By Name(w610) -> ("Name"=w608:string, "Variant Data"=w609:variant)
        n517 = invoke class="VI" method="Ctrl Val.Set"(error in=w607, "Control Name"=w608, "Value"=w609) -> (error out=w606:errorcluster)  [unwired: 2 in, 4 out]
      }
      "error out 2" <- w585
    }
    frame #1 {
      w614 = ""
      w615 = FALSE ("kill")
      w611 = T3."Disabled and Grayed Out" ("Disabled")
      n518 = local write "Tab Control"(enum32{"Page 1", "Page 2", "Page 3", "Page 4"}."Page 1" ("Tab Control")) -> ()
      n519 = local write "Satellite Name"(w614) -> ()
      n520 = local write "Radio Mode"(TRUE ("Radio Mode")) -> ()
      n521 = local write "Type of DN"(w614) -> ()
      n522 = local write "dont write"(FALSE ("dont write")) -> ()
      n523 = local write "kill"(w615) -> ()
      n524 = property on="kill" class="Bool (strict)"("Value"=w615) -> ()  [unwired: 2 in, 2 out]
      n525 = local read "WebSDRDB"() -> (w619:string[][])
      n526 = Transpose 2D Array(2D array=w619) -> (transposed array=w620:string[][])
      n527 = Index Array(array=w620) -> (element=w621:string[])  [unwired: 2 in]
      n528 = property on="Cat Control" class="Bool (strict)"("DisabledEnum"=T3."Enabled" ("Disabled"), "Value"=FALSE ("Cat Control")) -> ()  [unwired: 2 in, 2 out]
      n529 = property on="ManualLatch" class="Bool"("DisabledEnum"=w611) -> ()  [unwired: 2 in, 2 out]
      n530 = property on="Truncate Left digits" class="DigNum (strict)"("DisabledEnum"=w611) -> ()  [unwired: 2 in, 2 out]
      n531 = property on="Downlink Freq. Man." class="DigNum (strict)"("DisabledEnum"=w611) -> ()  [unwired: 2 in, 2 out]
      n532 = property on="Downlink corr." class="Knob (strict)"("DisabledEnum"=w611) -> ()  [unwired: 2 in, 2 out]
      n533 = property on="Radio Mode" class="Bool (strict)"("DisabledEnum"=w611) -> ()  [unwired: 2 in, 2 out]
      n534 = property on="Downlink Freq." class="Str"("DisabledEnum"=w611) -> ()  [unwired: 2 in, 2 out]
      n535 = property on="Stop Cat Control" class="Bool"("DisabledEnum"=w611) -> ()  [unwired: 2 in, 2 out]
      n536 = property on="WebPages" class="Ring (strict)"("Strings []"=w621) -> ()  [unwired: 2 in, 2 out]
    }
    frame #2 {
      n537 = while {
        stop <- w624 stop-if-true
        w628 = u32 1 items=["Down/Press", "Down then Up", "Up/Release"] ("Action")
        w633 = "WebSDR" ("Such-String")
        n538 = local read "Window title"() -> (w623:string)
        n539 = node-c288() -> (w636:T7)  [unwired: 4 in]
        n540 = Match Pattern(string=w623, regular expression=w633) -> (match substring=w634:string)  [unwired: 1 in, 3 out]
        n541 = for {
          N: 20 -> [_]
          tunnel: 8 -> [w739]
          tunnel: [w739] -> w627 mode=indexing
          tunnel: w628 -> [w738]
          tunnel: [w738] -> w626 mode=indexing
        }
        n542 = call "Get Window RefNum.vi"("window name (\"\")"=w623) -> ("error out"=w631:errorcluster, "window refnum (NaWR)"=w632:T6)  [unwired: 7 in]
        n543 = Equal?(x=w634, y=w633) -> (x = y?=w625:bool)
        n544 = timed-loop {
          tunnel: w632 -> [w657]
          tunnel: w631 -> [w656]
          tunnel: w625 -> [w653]
          tunnel: w627 -> [w655]
          tunnel: w626 -> [w654]
          timing: w636 -> [_]
          timing-out: [_] -> w635
          tunnel: [FALSE] -> w622
          stop <- w647 stop-if-true
          n545 = local read "Downlink Freq."() -> (w638:string)
          n546 = call "String Changed__ogtk.vi"("String"=w638) -> ("Changed"=w637:bool)
          n547 = local read "Truncate Left digits"() -> (w649:i32)
          n548 = local read "Cat Control"() -> (w639:bool)
          n549 = local read "dont write"() -> (w642:bool)
          n550 = And(x=w637, y=w653) -> (x .and. y?=w640:bool)
          n551 = local read "MaOps"() -> (w641:bool)
          n552 = And(x=w639, y=w640) -> (x .and. y?=w644:bool)
          n553 = String Subset(string=w638, offset (0)=w649) -> (substring=w650:string)  [unwired: 1 in]
          n554 = Compound Arithmetic op=OR(w641, w644, w642) -> (w643:bool)
          n555 = case shown="True" w643 {
            tunnel: w657 -> [_ w673]
            tunnel: w656 -> [w659 w672]
            tunnel: [w659 w671] -> w658
            tunnel: w650 -> [_ w670]
            tunnel: w655 -> [_ w669]
            tunnel: w654 -> [_ w668]
            frame False {
            }
            frame True {
              w666 = T10 0 items=["no dialog", "OK message", "continue or stop message", "OK message + warnings", "continue/stop + warnings"] ("type of dialog (OK msg:1)")
              n556 = stacked-sequence {
                seq-local: [w684 _ _] -> [_ _ w726]
                tunnel: w673 -> [w681 _ _]
                tunnel: w672 -> [w677 _ _]
                tunnel: [w676 _ _] -> w671
                tunnel: [_ _ w726] -> w667
                tunnel: w670 -> [_ w698 _]
                tunnel: w669 -> [_ w691 _]
                tunnel: w668 -> [_ w690 _]
                frame #0 {
                  n557 = call "Show Window.vi"("error in (no error)"=w677, "window refnum (NaWR)"=w681) -> ("error out"=w678:errorcluster, "window refnum out"=w680:T6)  [unwired: 4 in]
                  n558 = call "Move Window to Top.vi"("error in (no error)"=w678, "activate? (T)"=TRUE ("activate? (F)"), "window refnum (NaWR)"=w680) -> ("error out"=w679:errorcluster, "window refnum out"=w682:T6)  [unwired: 3 in]
                  n559 = call "Get Window Rectangle.vi"("error in (no error)"=w679, "window refnum (NaWR)"=w682) -> ("error out"=w676:errorcluster, "window rect"=→"window rect 2":T2, "window refnum out"=w684:T6)  [unwired: 3 in]
                }
                frame #1 {
                  w688 = u32 1 items=["Down/Press", "Down then Up", "Up/Release"] ("Action")
                  w700 = u32 1 items=["Down/Press", "Down then Up", "Up/Release"] ("Action")
                  n560 = String To Byte Array(string=w698) -> (unsigned byte array=w687:u8[])
                  n561 = for {
                    tunnel: w687 -> [w719] mode=indexing
                    tunnel: [w718] -> w703 mode=indexing
                    tunnel: [w717] -> w702 mode=indexing
                    w717 = u32 1 items=["Down/Press", "Down then Up", "Up/Release"] ("Action")
                    n562 = Equal?(x=w719, y=u8 46 ("Extended Keaystrokes_original_control 2")) -> (x = y?=w722:bool)
                    n563 = Select(t=u8 190 ("Extended Keaystrokes_original_control 2"), s=w722, f=w719) -> (s? t:f=w718:u8)
                  }
                  n564 = Insert Into Array(array=w691, new element #1=u8 71 ("Virtual Key 2"), new element #2=w703, new element #3=u8 9 ("Extended Keaystrokes_original_control 2")) -> (w701:i32[])  [unwired: 1 in]
                  n565 = Insert Into Array(array=w690, new element #1=w688, new element #2=w702, new element #3=w700) -> (w695:u32[])  [unwired: 1 in]
                  n566 = Array Size(array=w695) -> (size(s)=w694:i32)
                  n567 = node-c288(i64 100 ("Period")) -> (w697:T7)  [unwired: 3 in]
                  n568 = Increment(x=w694) -> (x+1=w693:i32)
                  n569 = Increment(x=w693) -> (x+1=w692:i32)
                  n570 = timed-loop {
                    tunnel: w701 -> [w709] mode=indexing
                    tunnel: w695 -> [w710] mode=indexing
                    timing: w697 -> [_]
                    timing-out: [_] -> w696
                    tunnel: w692 -> [w707]
                    i -> [w708]
                    stop <- w705 stop-if-true
                    n571 = local read "Interrupt"() -> (w704:bool)
                    n572 = Equal?(x=w708, y=w707) -> (x = y?=w706:bool)
                    n573 = Or(x=w706, y=w704) -> (x .or. y?=w705:bool)
                    n574 = call "Simulate Keyboard.vi"("Action"=w710, "Virtual Key"=w709) -> ()  [unwired: 7 in, 1 out]
                  }
                  n575 = node-c288(w696) -> ()  [unwired: 1 out]
                }
                frame #2 {
                  n576 = node-c288() -> (w725:T7)  [unwired: 4 in]
                  n577 = timed-loop {
                    shift-right: [w728] -> _
                    shift-left: FALSE ("Time has Elapsed") -> [w727]
                    timing: w725 -> [_]
                    timing-out: [_] -> w724
                    stop <- w728 stop-if-true
                    n578 = call "Elapsed Time"("Time Target (s)"=0.5, "Reset"=w727) -> ("Time has Elapsed"=w728:bool)  [unwired: 10 in, 7 out]
                  }
                  n579 = node-c288(w724) -> ()  [unwired: 1 out]
                }
              }
              n580 = call "Show Window.vi"("window refnum (NaWR)"=w667) -> ("error out"=w663:errorcluster)  [unwired: 5 in, 1 out]
              n581 = local read "FocusCheck"() -> (w660:bool)
              n582 = Unbundle By Name(w663) -> ("status"=w661:bool)
              n583 = call <vilib>:"Clear Errors.vi"("error in (no error)"=w663) -> ("error out"=w665:errorcluster)  [unwired: 5 in, 1 out]
              n584 = And(x=w660, y=w661) -> (x .and. y?=w662:bool)
              n585 = case shown="True" w662 {
                tunnel: "There sems to be\nan issue focussing\nyour WebSDR!\n\nTry disengage and reangage" ("message") -> [_ w675]
                frame False {
                }
                frame True {
                  n586 = One Button Dialog(message=w675, button name ("OK")="Wilco") -> ()  [unwired: 1 out]
                }
              }
              n587 = call <vilib>:"Simple Error Handler.vi"("type of dialog (OK msg:1)"=w666, "error in (no error)"=w665) -> ()  [unwired: 3 in, 5 out]
            }
          }
          "error out" <- w658
          n588 = local read "StopCatProgramatically"() -> (w645:bool)
          n589 = property on="kill" class="Bool (strict)"() -> ("Value"=w651:bool)  [unwired: 2 in, 2 out]
          n590 = Or(x="Stop Cat Control", y=w651) -> (x .or. y?=w648:bool)
          n591 = Or(x=w645, y=w648) -> (x .or. y?=w647:bool)
        }
        n592 = node-c288(w635) -> ()  [unwired: 1 out]
        n593 = local write "StopCatProgramatically"(w622) -> ()
        n594 = property on="kill" class="Bool (strict)"() -> ("Value"=w624:bool)  [unwired: 2 in, 2 out]
      }
    }
    frame #3 {
      n595 = while {
        tunnel: errorcluster {"status"=FALSE, "code"=0, "source"=""} ("error in (no error)") -> [w753]
        tunnel: [TRUE] -> w740
        stop <- w751 stop-if-true
        n596 = Compound Arithmetic op=AND("slave1Killed", "slave3Killed", "slave4Killed") -> ()  [unwired: 1 out]
        n597 = control-ref of="iterCompleted"() -> (w750:refnum<vi>)
        n598 = property on="iterCompleted" class="Bool (strict)"("Value"="slave1Killed") -> ()  [unwired: 2 in, 2 out]
        n599 = local write "iterCompleted"("slave1Killed") -> ()
        n600 = call "Marquee.vi"("Indicator or ctrl to look up value change"=w750, "Iteration"="Numeric", "error in (no error)"=w753, "Text"="Closing WebSDR Cat-Control....") -> ("shutdown"=w752:bool)  [unwired: 6 in, 1 out]
        "shutdown in" <- w752
        n601 = Or(x=w752, y="slave1Killed") -> (x .or. y?=w751:bool)
        n602 = Wait (ms)(milliseconds to wait=u32 1000) -> ()  [unwired: 1 out]
      }
      n603 = local write "Radio Mode"(TRUE ("Radio Mode")) -> ()
      n604 = local write "slave1Killed"(TRUE ("slave1Killed")) -> ()
      n605 = property on="iterCompleted" class="Bool (strict)"("Value"=FALSE ("iterCompleted")) -> ()  [unwired: 2 in, 2 out]
      n606 = Stop(stop? (T)=w740) -> ()
    }
  }
  n607 = while {
    shift-right: [w766] -> _
    shift-left: _ -> [w767]
    tunnel: [TRUE] -> w8
    stop <- "kill" stop-if-true
    w762 = u32 16860 ("Text.Text Colors:Text Color")
    w758 = T11 0 items=["Beide", "String-Anfang", "String-Ende"] ("location (both)")
    n608 = Wait (ms)(milliseconds to wait=u32 1000) -> ()  [unwired: 1 out]
    n609 = local read "data"() -> (w759:string)
    n610 = Match Pattern(string=w759, regular expression="AZ" ("Regulärer Ausdruck")) -> (after substring=w777:string)  [unwired: 1 in, 3 out]
    n611 = Match Pattern(string=w759, regular expression="SN\"" ("Regulärer Ausdruck")) -> (after substring=w780:string)  [unwired: 1 in, 3 out]
    n612 = Match Pattern(string=w759, regular expression="DN" ("Regulärer Ausdruck")) -> (after substring=w779:string)  [unwired: 1 in, 3 out]
    n613 = Match Pattern(string=w759, regular expression="DM" ("Regulärer Ausdruck")) -> (after substring=w784:string)  [unwired: 1 in, 3 out]
    n614 = Match Pattern(string=w777, regular expression="EL" ("Regulärer Ausdruck")) -> (before substring=w788:string, after substring=w778:string)  [unwired: 1 in, 2 out]
    n615 = Match Pattern(string=w780, regular expression="\" " ("Regulärer Ausdruck")) -> (before substring=w790:string)  [unwired: 1 in, 3 out]
    n616 = Match Pattern(string=w779, regular expression=" " ("Regulärer Ausdruck")) -> (before substring=w782:string)  [unwired: 1 in, 3 out]
    n617 = Match Pattern(string=w784, regular expression=" " ("Regulärer Ausdruck")) -> (before substring=w785:string)  [unwired: 1 in, 3 out]
    n618 = local write "Type of DN"(w785) -> ()
    n619 = Match Pattern(string=w778, regular expression="DN" ("Regulärer Ausdruck")) -> (before substring=w786:string)  [unwired: 1 in, 3 out]
    n620 = call <vilib>:"Trim Whitespace.vi"("string"=w788, "location (both)"=w758) -> ("trimmed string"=→"Azimuth":string)
    n621 = call <vilib>:"Trim Whitespace.vi"("string"=w786, "location (both)"=w758) -> ("trimmed string"=→"Elevation":string)
    n622 = call <vilib>:"Trim Whitespace.vi"("string"=w790, "location (both)"=w758) -> ("trimmed string"=→"Satellite Name":string)
    n623 = case shown="True" "Radio Mode" {
      tunnel: w782 -> [w805 _]
      tunnel: [w801 w823] -> w766
      tunnel: ["Radio Automatic mode" "Radio Manual mode"] -> w781
      tunnel: w767 -> [_ w818]
      frame False {
        n624 = Fract/Exp String To Number(use system decimal point (T)=FALSE, string=w805) -> (number=w799:dbl)  [unwired: 2 in, 1 out]
        n625 = Divide(x=w799, y=1000.0) -> (x/y=w798:dbl)
        n626 = property on="Mode" class="Str"("Text.TextColor"=u32 16711680) -> ()  [unwired: 2 in, 2 out]
        n627 = property on="ManualLatch" class="Bool"("Visible"=FALSE ("Sichtbar")) -> ()  [unwired: 2 in, 2 out]
        n628 = property on="Downlink Freq." class="Str"("Visible"=TRUE) -> ()  [unwired: 2 in, 2 out]
        n629 = property on="Downlink Freq. Man." class="DigNum (strict)"("Visible"=FALSE) -> ()  [unwired: 2 in, 2 out]
        n630 = local read "Downlink corr."() -> (w807:dbl)
        n631 = local write "dont write"(TRUE ("dont write")) -> ()
        n632 = Add(x=w798, y=w807) -> (x+y=w802:dbl)
        n633 = Number To Fractional String(use system decimal point (T)=FALSE, number=w802, precision (6)=i16 2) -> (F-format string=w801:string)  [unwired: 1 in]
      }
      frame True {
        n634 = local read "Downlink corr."() -> (w820:dbl)
        n635 = property on="Mode" class="Str"("Text.TextColor"=u32 6618880) -> ()  [unwired: 2 in, 2 out]
        n636 = property on="ManualLatch" class="Bool"("Visible"=TRUE ("Sichtbar")) -> ()  [unwired: 2 in, 2 out]
        n637 = property on="Downlink Freq. Man." class="DigNum (strict)"("Visible"=TRUE) -> ()  [unwired: 2 in, 2 out]
        n638 = property on="Downlink Freq." class="Str"("Visible"=FALSE) -> ()  [unwired: 2 in, 2 out]
        n639 = Add(x="Downlink Freq. Man.", y=w820) -> (x+y=w814:dbl)
        n640 = Number To Fractional String(use system decimal point (T)=FALSE, number=w814, precision (6)=i16 2) -> (F-format string=w813:string)  [unwired: 1 in]
        n641 = case shown="False" "ManualLatch" {
          tunnel: [w828 w830] -> w823
          tunnel: w813 -> [_ w830]
          tunnel: w818 -> [w828 _]
          tunnel: [FALSE TRUE] -> w811
          frame False {
          }
          frame True {
          }
        }
        "MaOps" <- w811
        n642 = local write "dont write"(FALSE ("dont write")) -> ()
      }
    }
    "Mode" <- w781
    "Downlink Freq." <- w766
    n643 = property on="processes Box" class="CmbBox"() -> ("DisabledEnum"=w757:T3)  [unwired: 2 in, 2 out]
    n644 = call "I8 Changed__ogtk.vi"("I8"=w757) -> ("Changed"=w756:bool)
    n645 = call "Elapsed Time3"("Reset"=w756) -> ("Time has Elapsed"=w760:bool)  [unwired: 11 in, 7 out]
    n646 = case shown="True" w760 {
      frame False {
      }
      frame True {
        w794 = T3."Disabled and Grayed Out" ("Disabled")
        n647 = property on="FocusWebSDR" class="Bool"("DisabledEnum"=w794) -> ()  [unwired: 2 in, 2 out]
        n648 = property on="AddWebSDR" class="Bool"("DisabledEnum"=w794) -> ()  [unwired: 2 in, 2 out]
        n649 = property on="processes Box" class="CmbBox"("DisabledEnum"=w794) -> ()  [unwired: 2 in, 2 out]
      }
    }
    n650 = control-ref of="WebSDR Location / Name"() -> (w765:refnum<vi>)
    n651 = control-ref of="Truncate digits"() -> (w764:refnum<vi>)
    n652 = control-ref of="WebSDR URL"() -> (w763:refnum<vi>)
    n653 = property on="Property Node" class="Str"(reference=w765, "Text.TextColor"=w762) -> ()  [unwired: 1 in, 2 out]
    n654 = property on="Property Node" class="Str"(reference=w764, "Text.TextColor"=w762) -> ()  [unwired: 1 in, 2 out]
    n655 = property on="Property Node" class="Str"(reference=w763, "Text.TextColor"=w762) -> ()  [unwired: 1 in, 2 out]
  }
  n656 = local write "slave4Killed"(w8) -> ()
  "Title 2" <- "WebSDR Cat Control" ("Title 2")
  "Title 3" <- "WebSDR Cat Control" ("Title 3")
